vi "FA Values View.vi"(11 "Model in":refnum<class "Model.lvclass">) -> ()   [LabVIEW 2016, in "M1M3SupportEUI_Views.lvlib"]
uses:
  M1M3SupportEUI_Views.lvlib
  Model/Model.lvclass
  Typedefs/FA Data And Events.ctl
  SALLV_m1m3/DataTypes/ForceActuatorData.ctl
  SALLV_m1m3/DataTypes/logevent_ForceActuatorForceWarning.ctl
  SALLV_m1m3/DataTypes/logevent_ForceActuatorInfo.ctl
  SALLV_m1m3/DataTypes/logevent_ForceActuatorState.ctl
  SALLV_m1m3/DataTypes/logevent_ForceActuatorWarning.ctl
  SALLV_m1m3/DataTypes/logevent_AppliedAberrationForces.ctl
  SALLV_m1m3/DataTypes/logevent_AppliedAccelerationForces.ctl
  SALLV_m1m3/DataTypes/logevent_AppliedActiveOpticForces.ctl
  SALLV_m1m3/DataTypes/logevent_AppliedAzimuthForces.ctl
  SALLV_m1m3/DataTypes/logevent_AppliedBalanceForces.ctl
  SALLV_m1m3/DataTypes/logevent_AppliedCylinderForces.ctl
  SALLV_m1m3/DataTypes/logevent_AppliedElevationForces.ctl
  SALLV_m1m3/DataTypes/logevent_AppliedForces.ctl
  SALLV_m1m3/DataTypes/logevent_AppliedOffsetForces.ctl
  SALLV_m1m3/DataTypes/logevent_AppliedStaticForces.ctl
  SALLV_m1m3/DataTypes/logevent_AppliedThermalForces.ctl
  SALLV_m1m3/DataTypes/logevent_AppliedVelocityForces.ctl
  SALLV_m1m3/DataTypes/logevent_RejectedAberrationForces.ctl
  SALLV_m1m3/DataTypes/logevent_RejectedAccelerationForces.ctl
  SALLV_m1m3/DataTypes/logevent_RejectedActiveOpticForces.ctl
  SALLV_m1m3/DataTypes/logevent_RejectedAzimuthForces.ctl
  SALLV_m1m3/DataTypes/logevent_RejectedBalanceForces.ctl
  SALLV_m1m3/DataTypes/logevent_RejectedCylinderForces.ctl
  SALLV_m1m3/DataTypes/logevent_RejectedElevationForces.ctl
  SALLV_m1m3/DataTypes/logevent_RejectedForces.ctl
  SALLV_m1m3/DataTypes/logevent_RejectedOffsetForces.ctl
  SALLV_m1m3/DataTypes/logevent_RejectedStaticForces.ctl
  SALLV_m1m3/DataTypes/logevent_RejectedThermalForces.ctl
  SALLV_m1m3/DataTypes/logevent_RejectedVelocityForces.ctl
  SALLV_m1m3/DataTypes/logevent_ForceSetpointWarning.ctl
  M1M3 Support Events/M1M3 Support Events.lvclass/M1M3 Support Events.ctl
  M1M3 Support Events/M1M3 Support Events.lvclass
  <vilib>/Utility/Data Type/NI_Data Type.lvlib
  SALLV_m1m3/SALLV_m1m3.lvlib
  Typedefs/M1M3SupportEUI_TypeDefs.lvlib
panel:
  out "stop":bool
  in  "FA Data And Events":T1 {"ForceActuatorData"."Timestamp" format="%#_14f"}
  out "SingleValue":string
  out "239":string
  out "229":string
  out "219":string
  out "209":string
  out "238":string
  out "228":string
  out "218":string
  out "208":string
  out "237":string
  out "227":string
  out "217":string
  out "207":string
  out "236":string
  out "216":string
  out "235":string
  out "225":string
  out "215":string
  out "234":string
  out "224":string
  out "214":string
  out "243":string
  out "233":string
  out "223":string
  out "242":string
  out "232":string
  out "222":string
  out "212":string
  out "241":string
  out "231":string
  out "221":string
  out "211":string
  out "240":string
  out "230":string
  out "220":string
  out "210":string
  out "339":string
  out "329":string
  out "319":string
  out "309":string
  out "338":string
  out "328":string
  out "318":string
  out "308":string
  out "337":string
  out "327":string
  out "317":string
  out "307":string
  out "336":string
  out "326":string
  out "316":string
  out "306":string
  out "335":string
  out "325":string
  out "315":string
  out "305":string
  out "334":string
  out "324":string
  out "314":string
  out "304":string
  out "343":string
  out "333":string
  out "323":string
  out "313":string
  out "303":string
  out "342":string
  out "332":string
  out "322":string
  out "312":string
  out "302":string
  out "341":string
  out "331":string
  out "321":string
  out "311":string
  out "301":string
  out "340":string
  out "330":string
  out "320":string
  out "310":string
  out "439":string
  out "429":string
  out "419":string
  out "409":string
  out "438":string
  out "428":string
  out "418":string
  out "408":string
  out "437":string
  out "427":string
  out "417":string
  out "407":string
  out "436":string
  out "416":string
  out "435":string
  out "425":string
  out "415":string
  out "434":string
  out "424":string
  out "414":string
  out "443":string
  out "433":string
  out "423":string
  out "442":string
  out "432":string
  out "422":string
  out "412":string
  out "441":string
  out "431":string
  out "421":string
  out "411":string
  out "440":string
  out "430":string
  out "420":string
  out "410":string
  out "139":string
  out "129":string
  out "119":string
  out "109":string
  out "138":string
  out "128":string
  out "118":string
  out "108":string
  out "137":string
  out "127":string
  out "117":string
  out "107":string
  out "136":string
  out "126":string
  out "116":string
  out "106":string
  out "135":string
  out "125":string
  out "115":string
  out "105":string
  out "134":string
  out "124":string
  out "114":string
  out "104":string
  out "143":string
  out "133":string
  out "123":string
  out "113":string
  out "103":string
  out "142":string
  out "132":string
  out "122":string
  out "112":string
  out "102":string
  out "141":string
  out "131":string
  out "121":string
  out "111":string
  out "101":string
  out "140":string
  out "130":string
  out "120":string
  out "110":string
  out "Timestamp of Data being shown":timestamp
  in  "Data Type":string(combo)
  # "Force Actuators"
  # "0"
  # "1"
  # "2"
  # "3"
  # "4"
  # "5"
  # "6"
  # "7"
  # "8"
  # "9"
  # "100"
  # "110"
  # "120"
  # "130"
  # "140"
  # "200"
  # "210"
  # "220"
  # "230"
  # "240"
  # "300"
  # "310"
  # "320"
  # "330"
  # "340"
  # "400"
  # "410"
  # "420"
  # "430"
  # "440"
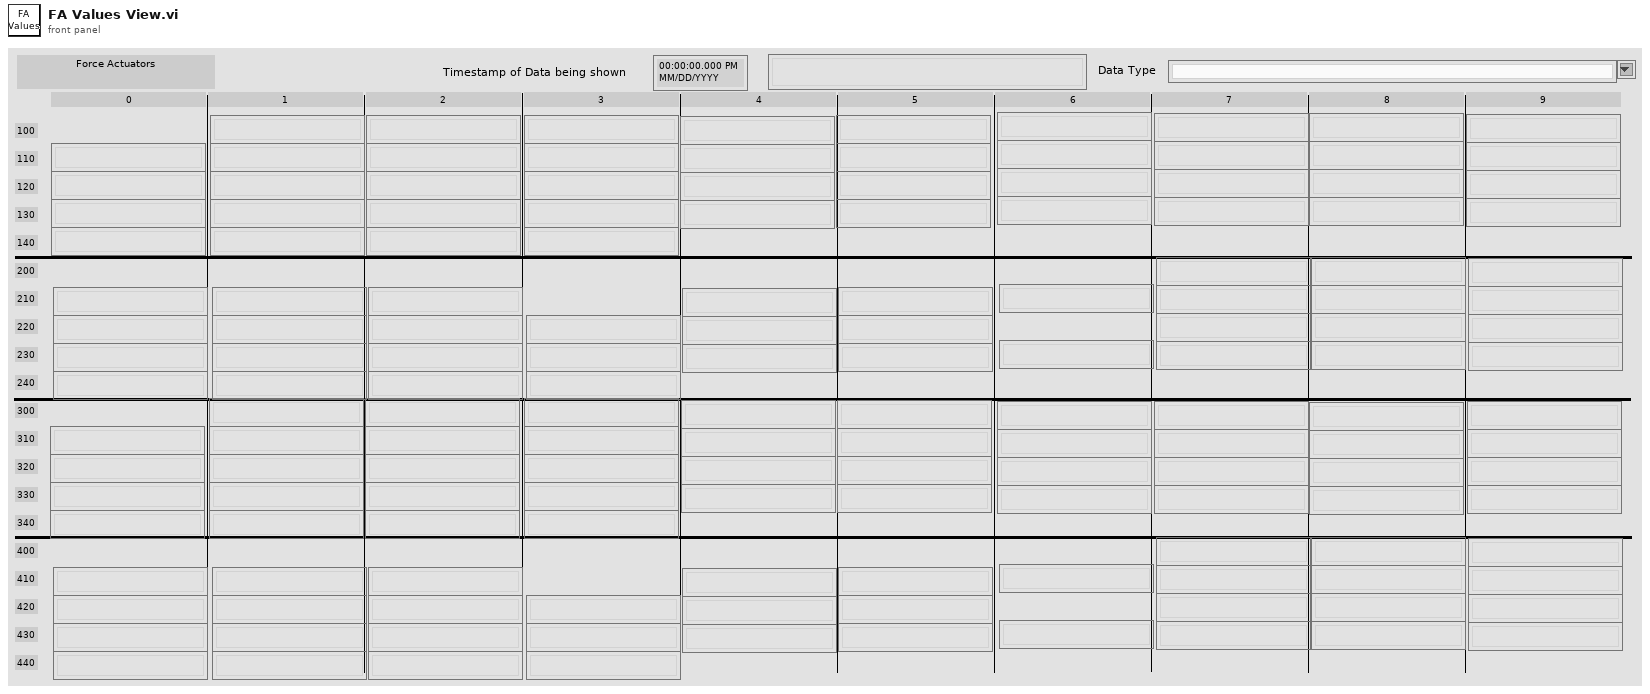
[diagram p1: front panel]
types:
  T1 = typedef "M1M3SupportEUI_TypeDefs.lvlib/FA Data And Events.ctl" = cluster{"ForceActuatorData":T2, "logevent_ForceActuatorForceWarning":T3, "logevent_ForceActuatorInfo":T4, "logevent_ForceActuatorState":T5, "logevent_ForceActuatorWarning":T6, "logevent_AppliedAberrationForces":T7, "logevent_AppliedAccelerationForces":T8, "logevent_AppliedActiveOpticForces":T9, "logevent_AppliedAzimuthForces":T10, "logevent_AppliedBalanceForces":T11, "logevent_AppliedCylinderForces":T12, "logevent_AppliedElevationForces":T13, "logevent_AppliedForces":T14, "logevent_AppliedOffsetForces":T15, "logevent_AppliedStaticForces":T16, "logevent_AppliedThermalForces":T17, "logevent_AppliedVelocityForces":T18, "logevent_RejectedAberrationForces":T19, "logevent_RejectedAccelerationForces":T20, "logevent_RejectedActiveOpticForces":T21, "logevent_RejectedAzimuthForces":T22, "logevent_RejectedBalanceForces":T23, "logevent_RejectedCylinderForces":T24, "logevent_RejectedElevationForces":T25, "logevent_RejectedForces":T26, "logevent_RejectedOffsetForces":T27, "logevent_RejectedStaticForces":T28, "logevent_RejectedThermalForces":T29, "logevent_RejectedVelocityForces":T30, "logevent_ForceSetpointWarning":T31}
  T2 = typedef "SALLV_m1m3.lvlib/ForceActuatorData.ctl" = cluster{"Timestamp":dbl, "PrimaryCylinderForce[156]":sgl[], "SecondaryCylinderForce[112]":sgl[], "XForce[12]":sgl[], "YForce[100]":sgl[], "ZForce[156]":sgl[], "Fx":sgl, "Fy":sgl, "Fz":sgl, "Mx":sgl, "My":sgl, "Mz":sgl, "ForceMagnitude":sgl}
  T3 = typedef "SALLV_m1m3.lvlib/logevent_ForceActuatorForceWarning.ctl" = cluster{"Timestamp":dbl, "AnyWarning":bool, "AnyPrimaryAxisMeasuredForceWarning":bool, "PrimaryAxisMeasuredForceWarning[156]":bool[], "AnySecondaryAxisMeasuredForceWarning":bool, "SecondaryAxisMeasuredForceWarning[156]":bool[], "AnyPrimaryAxisFollowingErrorWarning":bool, "PrimaryAxisFollowingErrorWarning[156]":bool[], "AnySecondaryAxisFollowingErrorWarning":bool, "SecondaryAxisFollowingErrorWarning[156]":bool[], "priority":i32}
  T4 = typedef "SALLV_m1m3.lvlib/logevent_ForceActuatorInfo.ctl" = cluster{"Timestamp":dbl, "ReferenceId[156]":i16[], "XDataReferenceId[12]":i16[], "YDataReferenceId[100]":i16[], "ZDataReferenceId[156]":i16[], "ActuatorType[156]":i16[], "ActuatorOrientation[156]":i16[], "ModbusSubnet[156]":i16[], "ModbusAddress[156]":i16[], "XPosition[156]":sgl[], "YPosition[156]":sgl[], "ZPosition[156]":sgl[], "ILCUniqueId[156]":i64[], "ILCApplicationType[156]":i16[], "NetworkNodeType[156]":i16[], "ILCSelectedOptions[156]":i16[], "NetworkNodeOptions[156]":i16[], "MajorRevision[156]":i16[], "MinorRevision[156]":i16[], "ADCScanRate[156]":i16[], "MainPrimaryCylinderCoefficient[156]":sgl[], "MainSecondaryCylinderCoefficient[156]":sgl[], "MainPrimaryCylinderLoadCellOffset[156]":sgl[], "MainSecondaryCylinderLoadCellOffset[156]":sgl[], "MainPrimaryCylinderLoadCellSensitivity[156]":sgl[], "MainSecondaryCylinderLoadCellSensitivity[156]":sgl[], "BackupPrimaryCylinderCoefficient[156]":sgl[], "BackupSecondaryCylinderCoefficient[156]":sgl[], "BackupPrimaryCylinderLoadCellOffset[156]":sgl[], "BackupSecondaryCylinderLoadCellOffset[156]":sgl[], "BackupPrimaryCylinderLoadCellSensitivity[156]":sgl[], "BackupSecondaryCylinderLoadCellSensitivity[156]":sgl[], "MezzaninePrimaryCylinderGain[156]":sgl[], "MezzanineSecondaryCylinderGain[156]":sgl[], "MezzanineUniqueId[156]":i64[], "MezzanineFirmwareType[156]":i16[], "MezzanineMajorRevision[156]":i16[], "MezzanineMinorRevision[156]":i16[], "priority":i32}
  T5 = typedef "SALLV_m1m3.lvlib/logevent_ForceActuatorState.ctl" = cluster{"Timestamp":dbl, "ILCState[156]":i16[], "SlewFlag":bool, "StaticForcesApplied":bool, "ElevationForcesApplied":bool, "AzimuthForcesApplied":bool, "ThermalForcesApplied":bool, "OffsetForcesApplied":bool, "AccelerationForcesApplied":bool, "VelocityForcesApplied":bool, "ActiveOpticForcesApplied":bool, "AberrationForcesApplied":bool, "BalanceForcesApplied":bool, "SupportPercentage":sgl, "priority":i32}
  T6 = typedef "SALLV_m1m3.lvlib/logevent_ForceActuatorWarning.ctl" = cluster{"Timestamp":dbl, "AnyWarning":bool, "AnyMajorFault":bool, "MajorFault[156]":bool[], "AnyMinorFault":bool, "MinorFault[156]":bool[], "AnyFaultOverride":bool, "FaultOverride[156]":bool[], "AnyMainCalibrationError":bool, "MainCalibrationError[156]":bool[], "AnyBackupCalibrationError":bool, "BackupCalibrationError[156]":bool[], "AnyMezzanineError":bool, "MezzanineError[156]":bool[], "AnyMezzanineBootloaderActive":bool, "MezzanineBootloaderActive[156]":bool[], "AnyUniqueIdCRCError":bool, "UniqueIdCRCError[156]":bool[], "AnyApplicationTypeMismatch":bool, "ApplicationTypeMismatch[156]":bool[], "AnyApplicationMissing":bool, "ApplicationMissing[156]":bool[], "AnyApplicationCRCMismatch":bool, "ApplicationCRCMismatch[156]":bool[], "AnyOneWireMissing":bool, "OneWireMissing[156]":bool[], "AnyOneWire1Mismatch":bool, "OneWire1Mismatch[156]":bool[], "AnyOneWire2Mismatch":bool, "OneWire2Mismatch[156]":bool[], "AnyWatchdogReset":bool, "WatchdogReset[156]":bool[], "AnyBrownOut":bool, "BrownOut[156]":bool[], "AnyEventTrapReset":bool, "EventTrapReset[156]":bool[], "AnySSRPowerFault":bool, "SSRPowerFault[156]":bool[], "AnyAuxPowerFault":bool, "AuxPowerFault[156]":bool[], "AnyMezzaninePowerFault":bool, "MezzaninePowerFault[156]":bool[], "AnyMezzanineCurrentAmp1Fault":bool, "MezzanineCurrentAmp1Fault[156]":bool[], "AnyMezzanineCurrentAmp2Fault":bool, "MezzanineCurrentAmp2Fault[156]":bool[], "AnyMezzanineUniqueIdCRCError":bool, "MezzanineUniqueIdCRCError[156]":bool[], "AnyMezzanineMainCalibrationError":bool, "MezzanineMainCalibrationError[156]":bool[], "AnyMezzanineBackupCalibrationError":bool, "MezzanineBackupCalibrationError[156]":bool[], "AnyMezzanineEventTrapReset":bool, "MezzanineEventTrapReset[156]":bool[], "AnyMezzanineApplicationMissing":bool, "MezzanineApplicationMissing[156]":bool[], "AnyMezzanineApplicationCRCMismatch":bool, "MezzanineApplicationCRCMismatch[156]":bool[], "AnyILCFault":bool, "ILCFault[156]":bool[], "AnyBroadcastCounterWarning":bool, "BroadcastCounterWarning[156]":bool[], "priority":i32}
  T7 = typedef "SALLV_m1m3.lvlib/logevent_AppliedAberrationForces.ctl" = cluster{"Timestamp":dbl, "ZForces[156]":sgl[], "Fz":sgl, "Mx":sgl, "My":sgl, "priority":i32}
  T8 = typedef "SALLV_m1m3.lvlib/logevent_AppliedAccelerationForces.ctl" = cluster{"Timestamp":dbl, "XForces[12]":sgl[], "YForces[100]":sgl[], "ZForces[156]":sgl[], "Fx":sgl, "Fy":sgl, "Fz":sgl, "Mx":sgl, "My":sgl, "Mz":sgl, "ForceMagnitude":sgl, "priority":i32}
  T9 = typedef "SALLV_m1m3.lvlib/logevent_AppliedActiveOpticForces.ctl" = cluster{"Timestamp":dbl, "ZForces[156]":sgl[], "Fz":sgl, "Mx":sgl, "My":sgl, "priority":i32}
  T10 = typedef "SALLV_m1m3.lvlib/logevent_AppliedAzimuthForces.ctl" = cluster{"Timestamp":dbl, "XForces[12]":sgl[], "YForces[100]":sgl[], "ZForces[156]":sgl[], "Fx":sgl, "Fy":sgl, "Fz":sgl, "Mx":sgl, "My":sgl, "Mz":sgl, "ForceMagnitude":sgl, "priority":i32}
  T11 = typedef "SALLV_m1m3.lvlib/logevent_AppliedBalanceForces.ctl" = cluster{"Timestamp":dbl, "XForces[12]":sgl[], "YForces[100]":sgl[], "ZForces[156]":sgl[], "Fx":sgl, "Fy":sgl, "Fz":sgl, "Mx":sgl, "My":sgl, "Mz":sgl, "ForceMagnitude":sgl, "priority":i32}
  T12 = typedef "SALLV_m1m3.lvlib/logevent_AppliedCylinderForces.ctl" = cluster{"Timestamp":dbl, "SecondaryCylinderForces[112]":i32[], "PrimaryCylinderForces[156]":i32[], "priority":i32}
  T13 = typedef "SALLV_m1m3.lvlib/logevent_AppliedElevationForces.ctl" = cluster{"Timestamp":dbl, "XForces[12]":sgl[], "YForces[100]":sgl[], "ZForces[156]":sgl[], "Fx":sgl, "Fy":sgl, "Fz":sgl, "Mx":sgl, "My":sgl, "Mz":sgl, "ForceMagnitude":sgl, "priority":i32}
  T14 = typedef "SALLV_m1m3.lvlib/logevent_AppliedForces.ctl" = cluster{"Timestamp":dbl, "XForces[12]":sgl[], "YForces[100]":sgl[], "ZForces[156]":sgl[], "Fx":sgl, "Fy":sgl, "Fz":sgl, "Mx":sgl, "My":sgl, "Mz":sgl, "ForceMagnitude":sgl, "priority":i32}
  T15 = typedef "SALLV_m1m3.lvlib/logevent_AppliedOffsetForces.ctl" = cluster{"Timestamp":dbl, "XForces[12]":sgl[], "YForces[100]":sgl[], "ZForces[156]":sgl[], "Fx":sgl, "Fy":sgl, "Fz":sgl, "Mx":sgl, "My":sgl, "Mz":sgl, "ForceMagnitude":sgl, "priority":i32}
  T16 = typedef "SALLV_m1m3.lvlib/logevent_AppliedStaticForces.ctl" = cluster{"Timestamp":dbl, "XForces[12]":sgl[], "YForces[100]":sgl[], "ZForces[156]":sgl[], "Fx":sgl, "Fy":sgl, "Fz":sgl, "Mx":sgl, "My":sgl, "Mz":sgl, "ForceMagnitude":sgl, "priority":i32}
  T17 = typedef "SALLV_m1m3.lvlib/logevent_AppliedThermalForces.ctl" = cluster{"Timestamp":dbl, "XForces[12]":sgl[], "YForces[100]":sgl[], "ZForces[156]":sgl[], "Fx":sgl, "Fy":sgl, "Fz":sgl, "Mx":sgl, "My":sgl, "Mz":sgl, "ForceMagnitude":sgl, "priority":i32}
  T18 = typedef "SALLV_m1m3.lvlib/logevent_AppliedVelocityForces.ctl" = cluster{"Timestamp":dbl, "XForces[12]":sgl[], "YForces[100]":sgl[], "ZForces[156]":sgl[], "Fx":sgl, "Fy":sgl, "Fz":sgl, "Mx":sgl, "My":sgl, "Mz":sgl, "ForceMagnitude":sgl, "priority":i32}
  T19 = typedef "SALLV_m1m3.lvlib/logevent_RejectedAberrationForces.ctl" = cluster{"Timestamp":dbl, "ZForces[156]":sgl[], "Fz":sgl, "Mx":sgl, "My":sgl, "priority":i32}
  T20 = typedef "SALLV_m1m3.lvlib/logevent_RejectedAccelerationForces.ctl" = cluster{"Timestamp":dbl, "XForces[12]":sgl[], "YForces[100]":sgl[], "ZForces[156]":sgl[], "Fx":sgl, "Fy":sgl, "Fz":sgl, "Mx":sgl, "My":sgl, "Mz":sgl, "ForceMagnitude":sgl, "priority":i32}
  T21 = typedef "SALLV_m1m3.lvlib/logevent_RejectedActiveOpticForces.ctl" = cluster{"Timestamp":dbl, "ZForces[156]":sgl[], "Fz":sgl, "Mx":sgl, "My":sgl, "priority":i32}
  T22 = typedef "SALLV_m1m3.lvlib/logevent_RejectedAzimuthForces.ctl" = cluster{"Timestamp":dbl, "XForces[12]":sgl[], "YForces[100]":sgl[], "ZForces[156]":sgl[], "Fx":sgl, "Fy":sgl, "Fz":sgl, "Mx":sgl, "My":sgl, "Mz":sgl, "ForceMagnitude":sgl, "priority":i32}
  T23 = typedef "SALLV_m1m3.lvlib/logevent_RejectedBalanceForces.ctl" = cluster{"Timestamp":dbl, "XForces[12]":sgl[], "YForces[100]":sgl[], "ZForces[156]":sgl[], "Fx":sgl, "Fy":sgl, "Fz":sgl, "Mx":sgl, "My":sgl, "Mz":sgl, "ForceMagnitude":sgl, "priority":i32}
  T24 = typedef "SALLV_m1m3.lvlib/logevent_RejectedCylinderForces.ctl" = cluster{"Timestamp":dbl, "SecondaryCylinderForces[112]":i32[], "PrimaryCylinderForces[156]":i32[], "priority":i32}
  T25 = typedef "SALLV_m1m3.lvlib/logevent_RejectedElevationForces.ctl" = cluster{"Timestamp":dbl, "XForces[12]":sgl[], "YForces[100]":sgl[], "ZForces[156]":sgl[], "Fx":sgl, "Fy":sgl, "Fz":sgl, "Mx":sgl, "My":sgl, "Mz":sgl, "ForceMagnitude":sgl, "priority":i32}
  T26 = typedef "SALLV_m1m3.lvlib/logevent_RejectedForces.ctl" = cluster{"Timestamp":dbl, "XForces[12]":sgl[], "YForces[100]":sgl[], "ZForces[156]":sgl[], "Fx":sgl, "Fy":sgl, "Fz":sgl, "Mx":sgl, "My":sgl, "Mz":sgl, "ForceMagnitude":sgl, "priority":i32}
  T27 = typedef "SALLV_m1m3.lvlib/logevent_RejectedOffsetForces.ctl" = cluster{"Timestamp":dbl, "XForces[12]":sgl[], "YForces[100]":sgl[], "ZForces[156]":sgl[], "Fx":sgl, "Fy":sgl, "Fz":sgl, "Mx":sgl, "My":sgl, "Mz":sgl, "ForceMagnitude":sgl, "priority":i32}
  T28 = typedef "SALLV_m1m3.lvlib/logevent_RejectedStaticForces.ctl" = cluster{"Timestamp":dbl, "XForces[12]":sgl[], "YForces[100]":sgl[], "ZForces[156]":sgl[], "Fx":sgl, "Fy":sgl, "Fz":sgl, "Mx":sgl, "My":sgl, "Mz":sgl, "ForceMagnitude":sgl, "priority":i32}
  T29 = typedef "SALLV_m1m3.lvlib/logevent_RejectedThermalForces.ctl" = cluster{"Timestamp":dbl, "XForces[12]":sgl[], "YForces[100]":sgl[], "ZForces[156]":sgl[], "Fx":sgl, "Fy":sgl, "Fz":sgl, "Mx":sgl, "My":sgl, "Mz":sgl, "ForceMagnitude":sgl, "priority":i32}
  T30 = typedef "SALLV_m1m3.lvlib/logevent_RejectedVelocityForces.ctl" = cluster{"Timestamp":dbl, "XForces[12]":sgl[], "YForces[100]":sgl[], "ZForces[156]":sgl[], "Fx":sgl, "Fy":sgl, "Fz":sgl, "Mx":sgl, "My":sgl, "Mz":sgl, "ForceMagnitude":sgl, "priority":i32}
  T31 = typedef "SALLV_m1m3.lvlib/logevent_ForceSetpointWarning.ctl" = cluster{"Timestamp":dbl, "AnyWarning":bool, "AnySafetyLimitWarning":bool, "SafetyLimitWarning[156]":bool[], "XMomentWarning":bool, "YMomentWarning":bool, "ZMomentWarning":bool, "AnyNearNeighborWarning":bool, "NearNeighborWarning[156]":bool[], "MagnitudeWarning":bool, "AnyFarNeighborWarning":bool, "FarNeighborWarning[156]":bool[], "AnyElevationForceWarning":bool, "ElevationForceWarning[156]":bool[], "AnyAzimuthForceWarning":bool, "AzimuthForceWarning[156]":bool[], "AnyThermalForceWarning":bool, "ThermalForceWarning[156]":bool[], "AnyBalanceForceWarning":bool, "BalanceForceWarning[156]":bool[], "AnyAccelerationForceWarning":bool, "AccelerationForceWarning[156]":bool[], "ActiveOpticNetForceWarning":bool, "AnyActiveOpticForceWarning":bool, "ActiveOpticForceWarning[156]":bool[], "AnyStaticForceWarning":bool, "StaticForceWarning[156]":bool[], "AberrationNetForceWarning":bool, "AnyAberrationForceWarning":bool, "AberrationForceWarning[156]":bool[], "AnyOffsetForceWarning":bool, "OffsetForceWarning[156]":bool[], "AnyVelocityForceWarning":bool, "VelocityForceWarning[156]":bool[], "AnyForceWarning":bool, "ForceWarning[156]":bool[], "priority":i32}
  T32 = typedef "M1M3SupportEUI_TypeDefs.lvlib/M1M3 Support Events.ctl" = cluster{"Inclinometer  Data":refnum<user-event>, "IMS Data":refnum<user-event>, "SAL Connected":refnum<user-event>, "Accelerometer Data":refnum<user-event>, "OuterLoop Data":refnum<user-event>, "ErrorCode Event":refnum<user-event>, "InterlockStatus Event":refnum<user-event>, "InterlockWarning Event":refnum<user-event>, "Gyro Data":refnum<user-event>, "HP Actuator Info Event":refnum<user-event>, " FA Info Event":refnum<user-event>, "HP Monitor Info Event":refnum<user-event>, "FA Data":refnum<user-event>, "HP Actuator data":refnum<user-event>, "HP Monitor data":refnum<user-event>, "Air Supply Status Event":refnum<user-event>, "Air Supply Warning Event":refnum<user-event>, "Power Data":refnum<user-event>, "PID Data":refnum<user-event>, "PID Info Event":refnum<user-event>, "Power Status Event":refnum<user-event>, "Power Supply Status Event":refnum<user-event>, "Power Warning Event":refnum<user-event>, "Summary State Event":refnum<user-event>, "Detailed State Event":refnum<user-event>, "FA Force Warning Event":refnum<user-event>, "FA Warning Event":refnum<user-event>, "FA State Event":refnum<user-event>, "Applied AberrationForces Event":refnum<user-event>, "Applied Acceleration Forcces Event":refnum<user-event>, "Applied Azimuth Forces Event":refnum<user-event>, "Applied Active Optic Forces Event":refnum<user-event>, "Applied Balance Forces Event":refnum<user-event>, "Applied Cylinder Forces Event":refnum<user-event>, "Applied Elevation Forces Event":refnum<user-event>, "Applied Forces Event":refnum<user-event>, "Applied Offset Forces Event":refnum<user-event>, "Applied Static Forces Event":refnum<user-event>, "Applied Thermal Forces Event":refnum<user-event>, "Applied Velocity Forces Event":refnum<user-event>, "Rejected Aberration Force Event":refnum<user-event>, "Rejected Acceleration Forces Event":refnum<user-event>, "Rejected Active Optic Forces Event":refnum<user-event>, "Rejected Azimuth Forces Event":refnum<user-event>, "Rejected Balance Forces Event":refnum<user-event>, "Rejected Cylinder Forces Event":refnum<user-event>, "Rejected Elevation Forces Event":refnum<user-event>, "Rejected Forces Event":refnum<user-event>, "Rejected Offset Forces Event":refnum<user-event>, "Rejected Static Forces Event":refnum<user-event>, "Rejected Thermal Forces Event":refnum<user-event>, "Rejected Velocity Forces Event":refnum<user-event>, "Command Rejection Event":refnum<user-event>, "Setting Verions Event":refnum<user-event>, "Settings Applied Event":refnum<user-event>, "HP Actuator State Event":refnum<user-event>, "HP Actuator Warning Event":refnum<user-event>, "HP Monitor State Event":refnum<user-event>, "HP Monitor Warning Event":refnum<user-event>, "Accelerometer Warning Event":refnum<user-event>, "Applied Settings Match Start Event":refnum<user-event>, "Cell Light Status Event ":refnum<user-event>, "Cell Light Warning Event":refnum<user-event>, "Displacement Sensor Warning Event":refnum<user-event>, "Force Setpoint Warning Event":refnum<user-event>, "Gyro Warning Event ":refnum<user-event>, "ILC Warning Event ":refnum<user-event>, "Inclinometer Sensor Warning Event ":refnum<user-event>}
  T33 = typedef "NI_Data Type.lvlib/Data Type.ctl" = enum8{"Invalid Type", "Void", "I8", "I16", "I32", "I64", "U8", "U16", "U32", "U64", "Single Float", "Double Float", "Extended Float", "Single Complex", "Double Complex", "Extended Complex", "Enum U8", "Enum U16", "Enum U32", "Enum U64", "Single Float With Unit", "Double Float With Unit", "Extended Float With Unit", "Single Complex with Unit", "Double Complex with Unit", "Extended Complex with Unit", "Boolean", "String", "Path", "Picture", "Tag", "Array", "Cluster", "Variant", "LV Variant", "Waveform", "Timestamp", "Digital Waveform", "Digital Data", "ExpressData", "Refnum", "External Data", "VI", "Poly VI", "LabVIEW Class Instance", "Fixed Point"}
  T34 = enum16{"", "DetailedState_DetailedStates_DisabledState", "DetailedState_DetailedStates_EnabledState", "DetailedState_DetailedStates_FaultState", "DetailedState_DetailedStates_OfflineState", "DetailedState_DetailedStates_StandbyState", "DetailedState_DetailedStates_ParkedState", "DetailedState_DetailedStates_RaisingState", "DetailedState_DetailedStates_ActiveState", "DetailedState_DetailedStates_LoweringState", "DetailedState_DetailedStates_EngineeringState", "DetailedState_DetailedStates_ParkedEngineeringState", "DetailedState_DetailedStates_RaisingEngineeringState", "DetailedState_DetailedStates_ActiveEngineeringState", "DetailedState_DetailedStates_LoweringEngineeringState", "DetailedState_DetailedStates_LoweringFaultState", "DetailedState_DetailedStates_ProfileHardpointCorrectionState"}
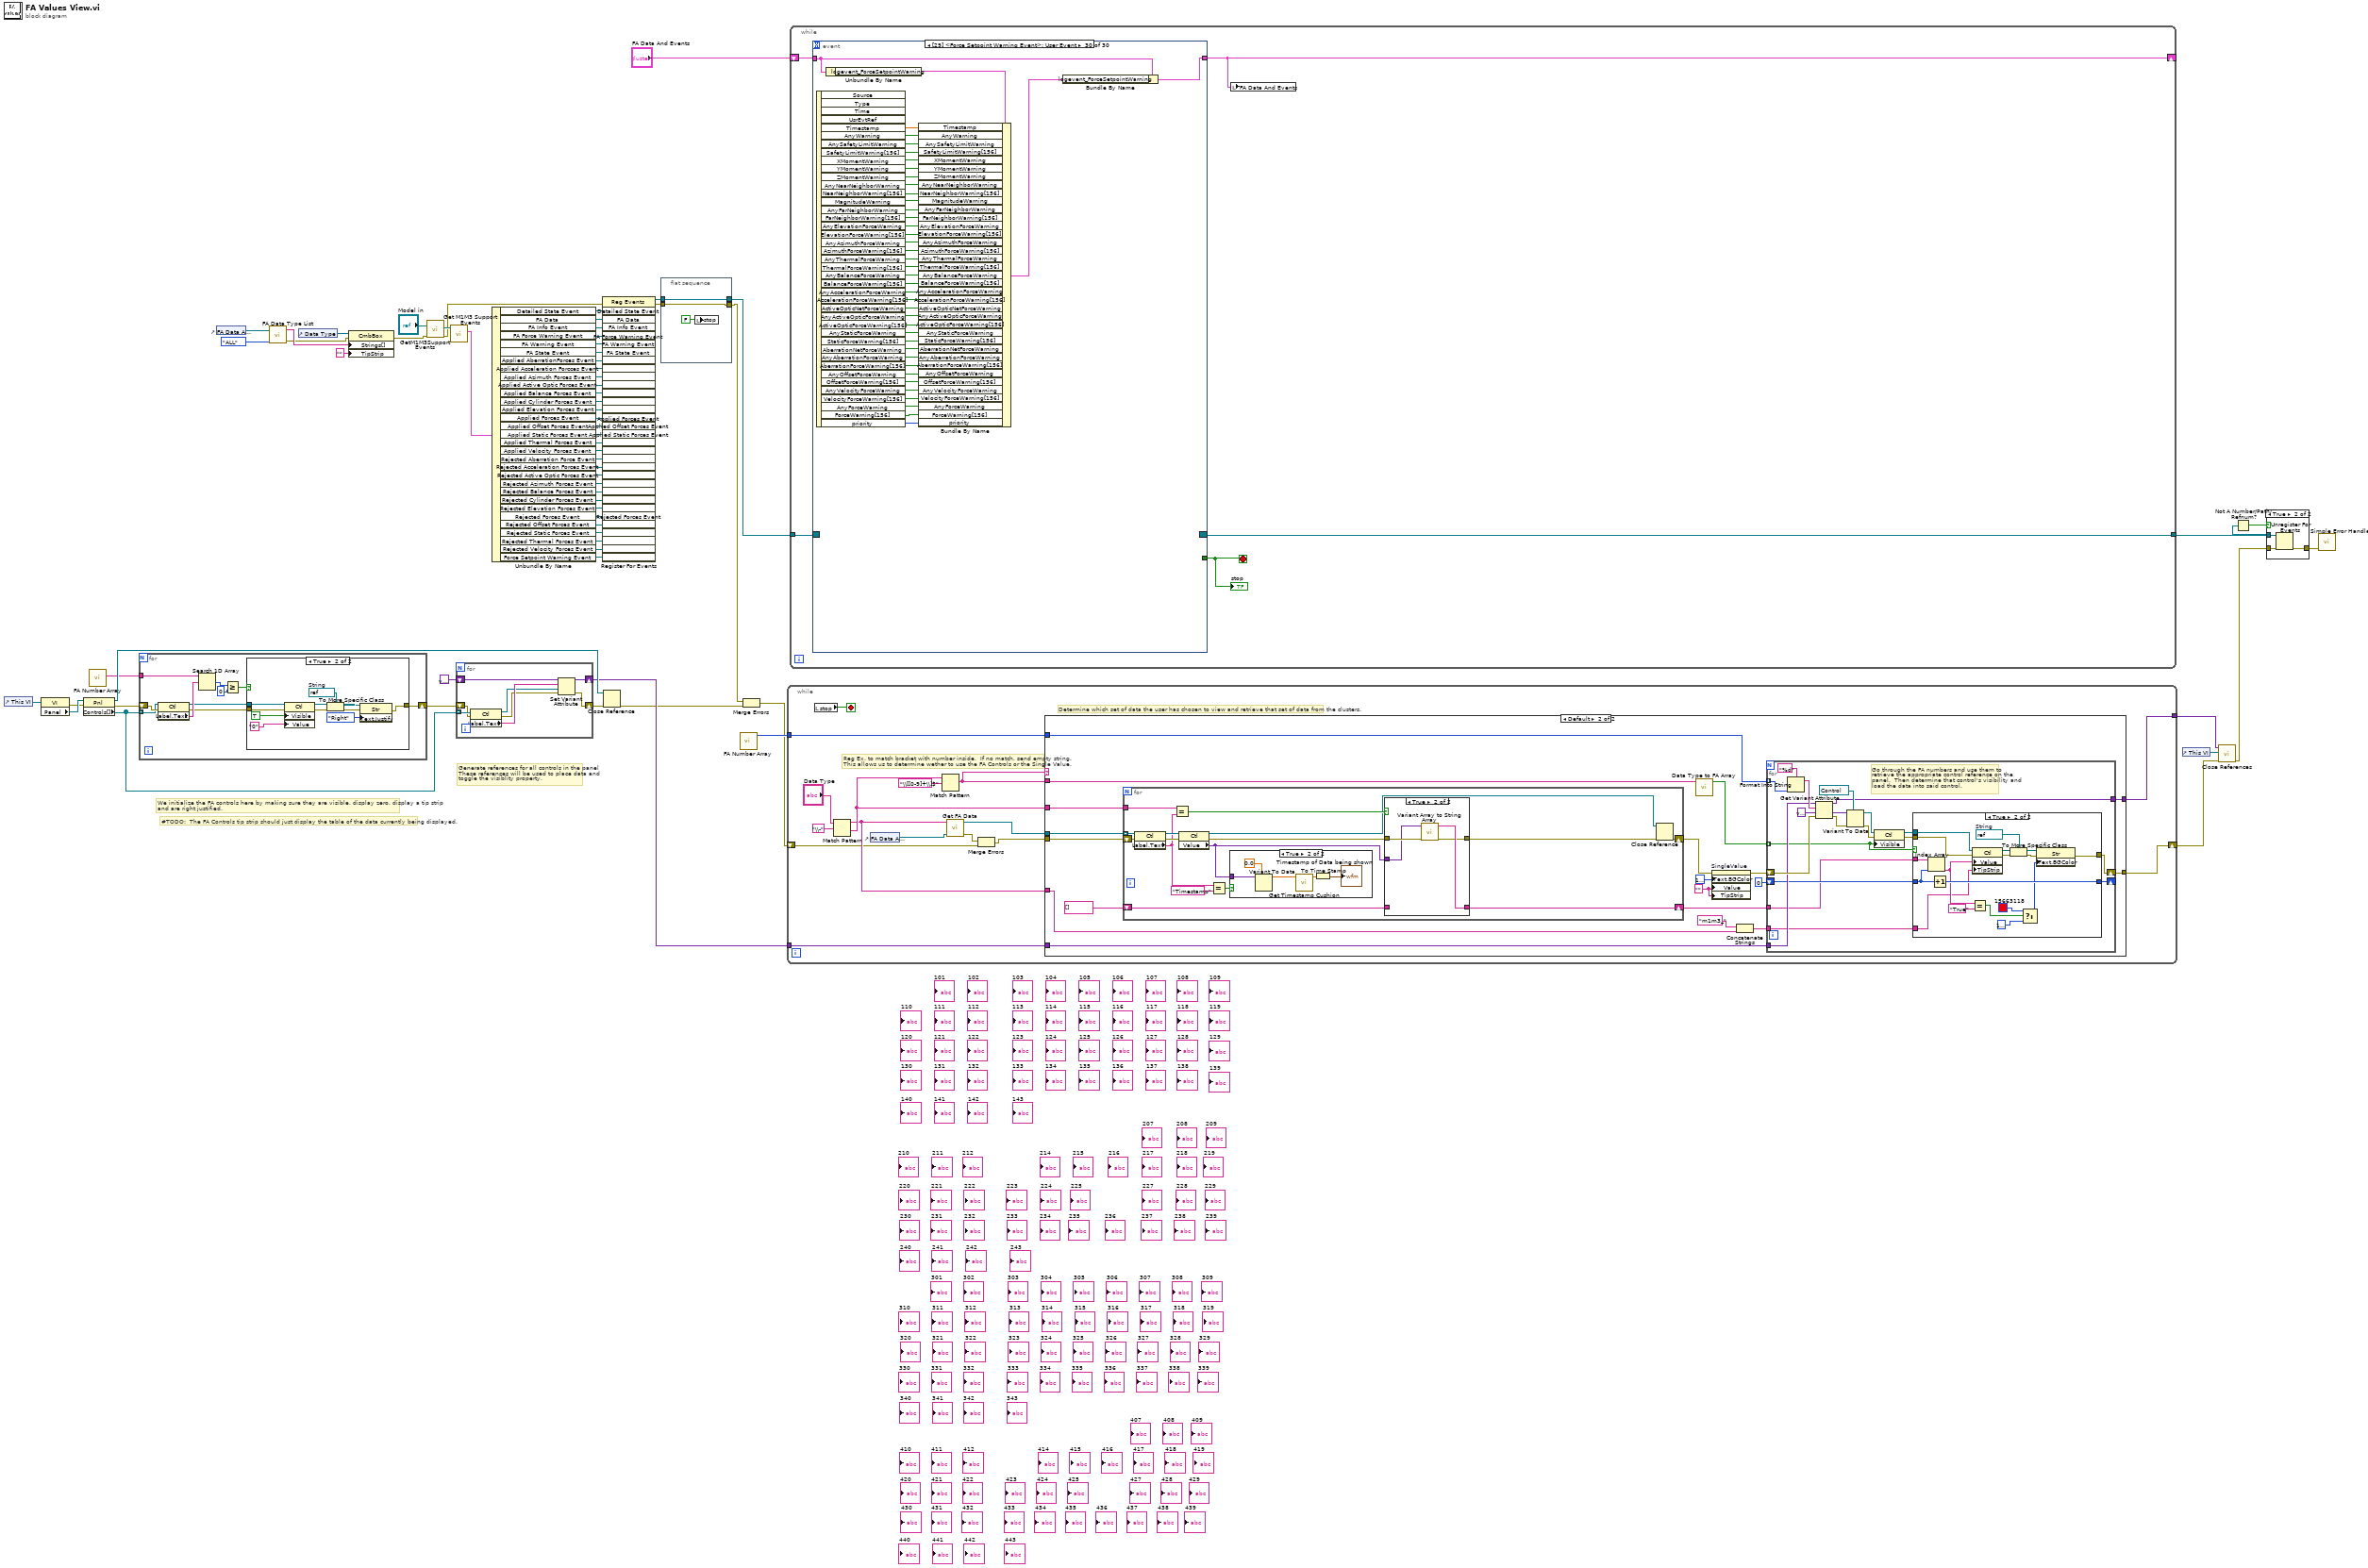
[diagram p0: block diagram]
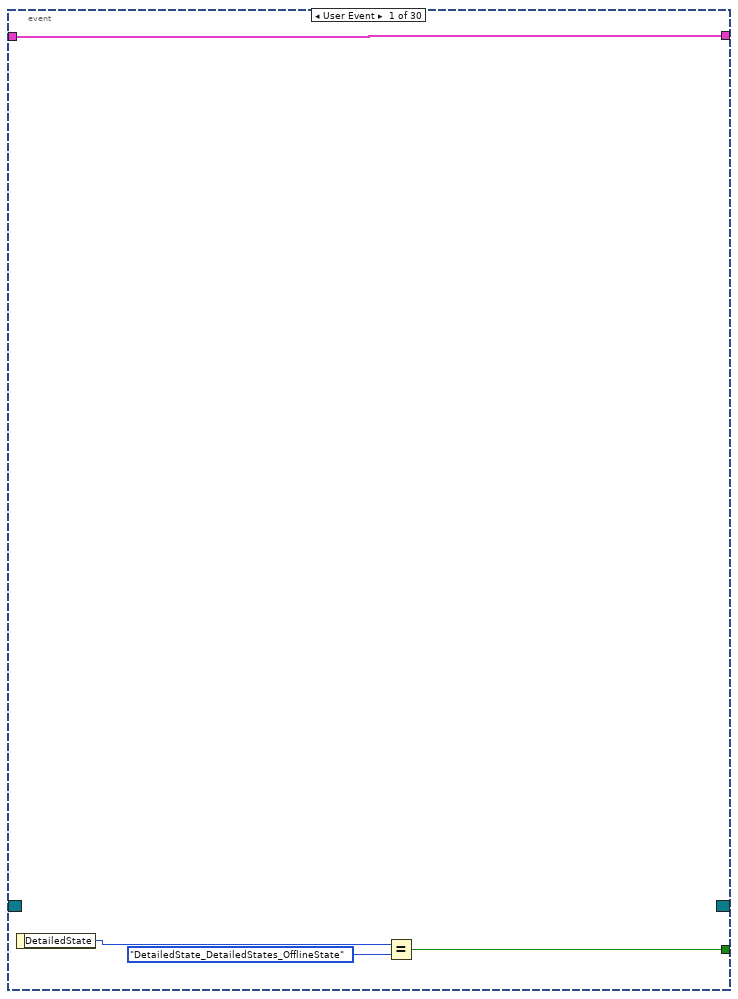
[diagram p3: hidden frame]
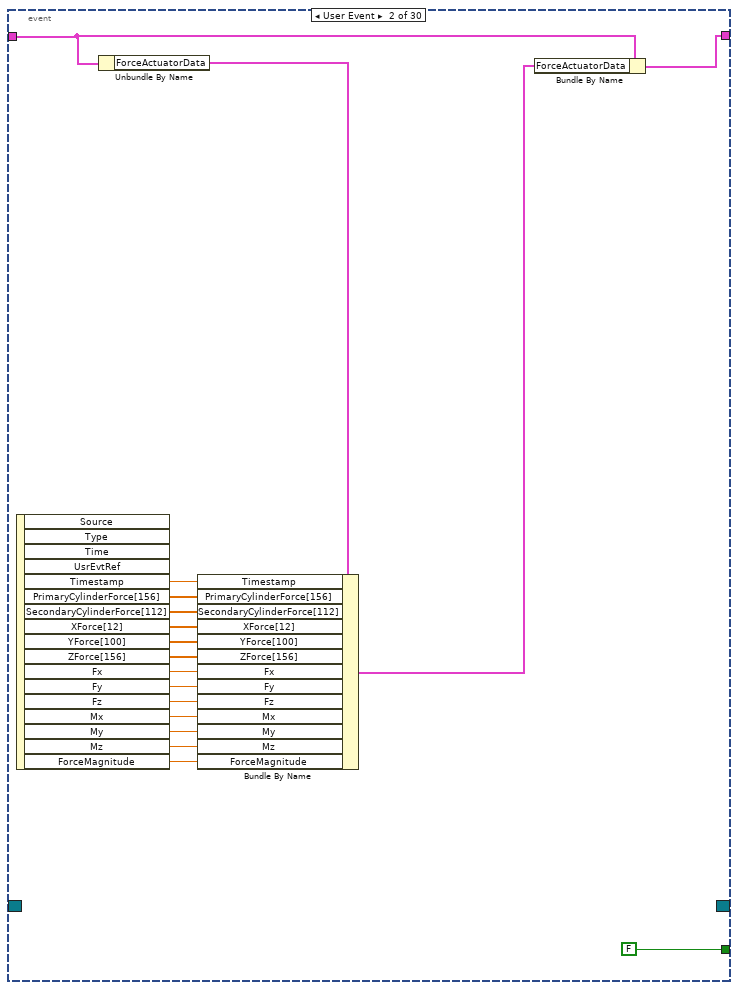
[diagram p4: hidden frame]
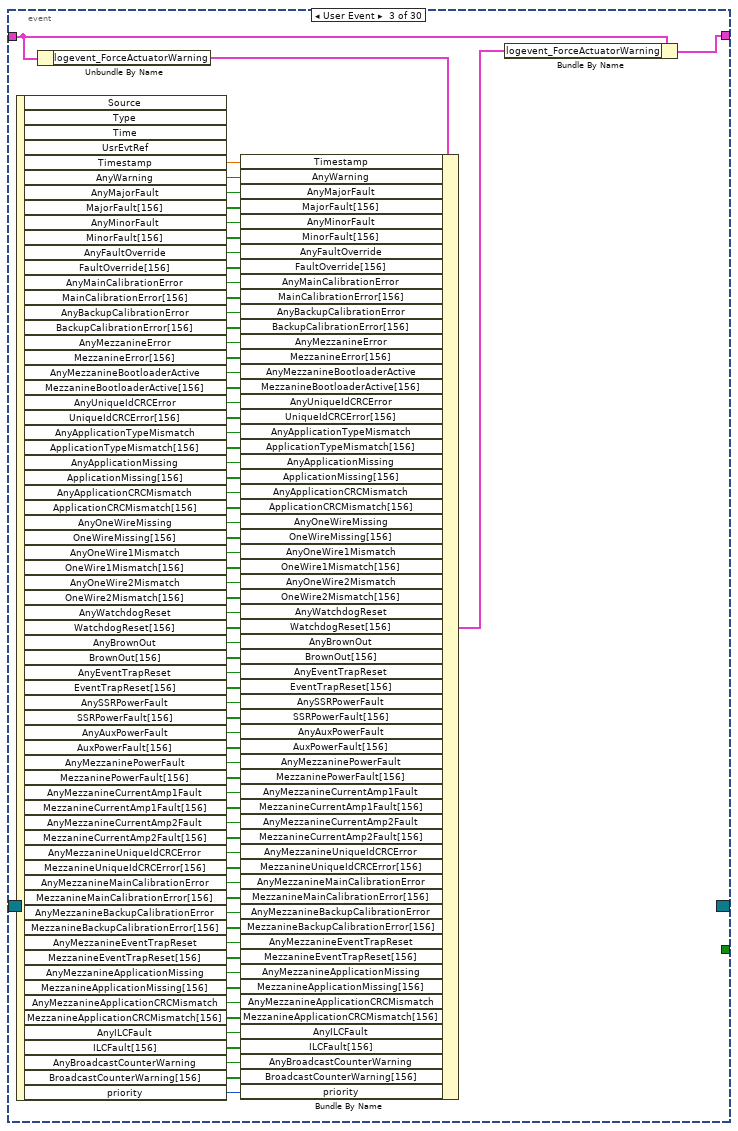
[diagram p5: hidden frame]
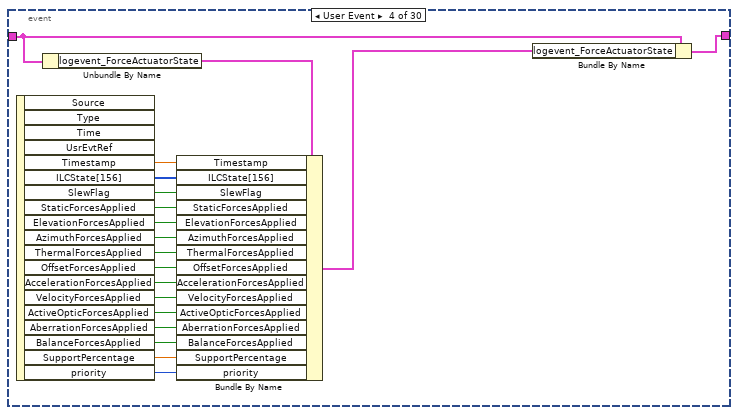
[diagram p6: hidden frame]
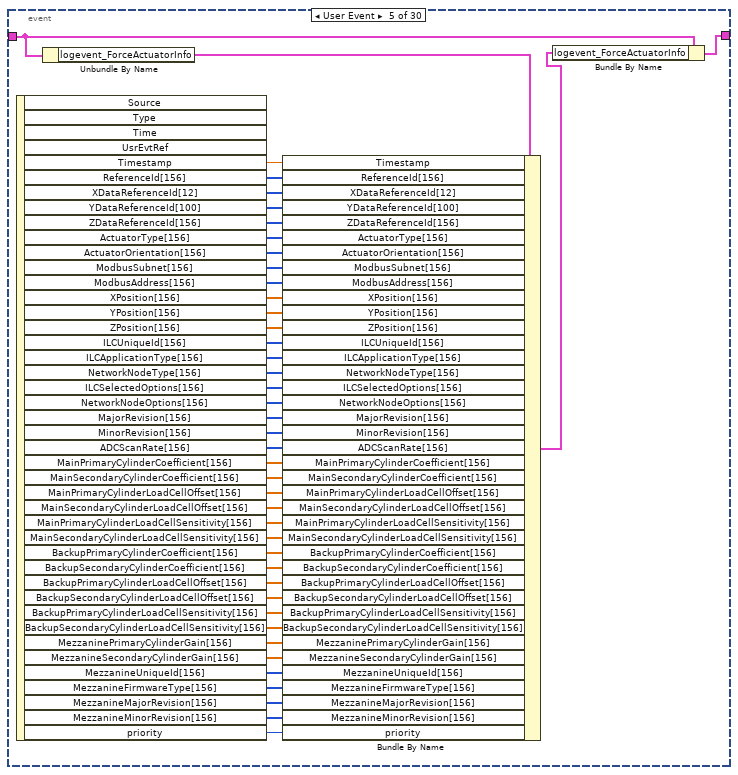
[diagram p7: hidden frame]
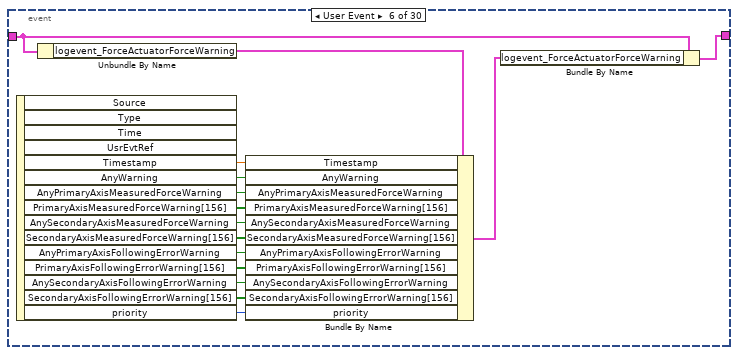
[diagram p8: hidden frame]
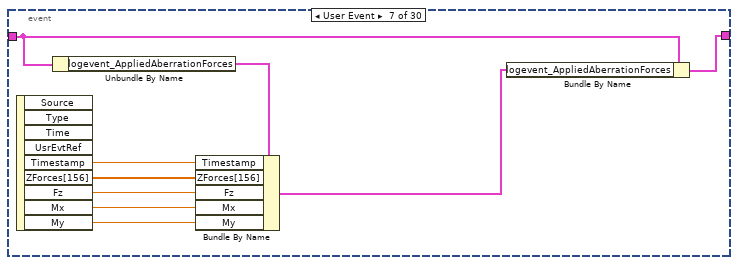
[diagram p9: hidden frame]
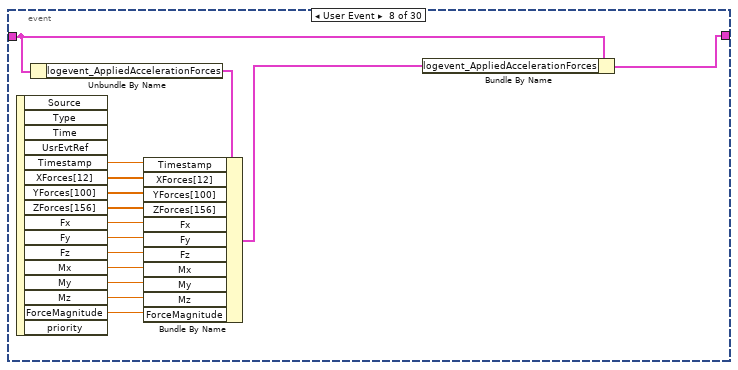
[diagram p10: hidden frame]
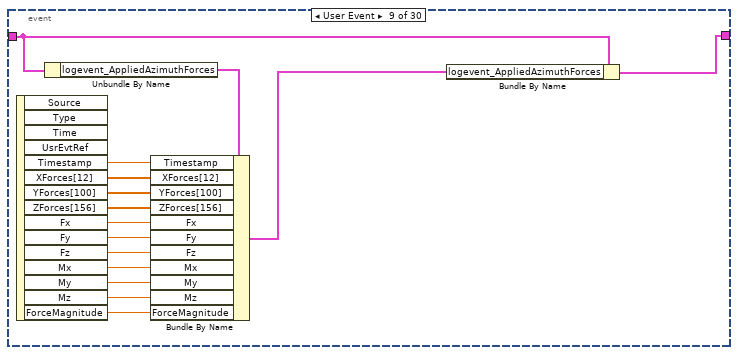
[diagram p11: hidden frame]
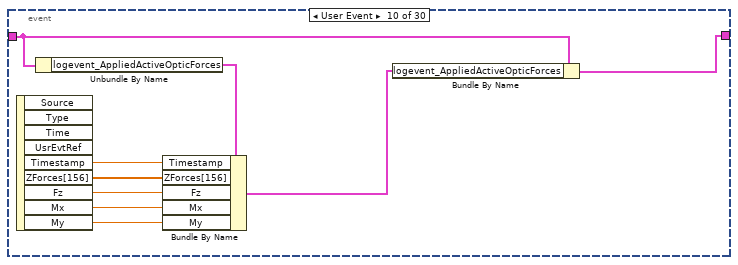
[diagram p12: hidden frame]
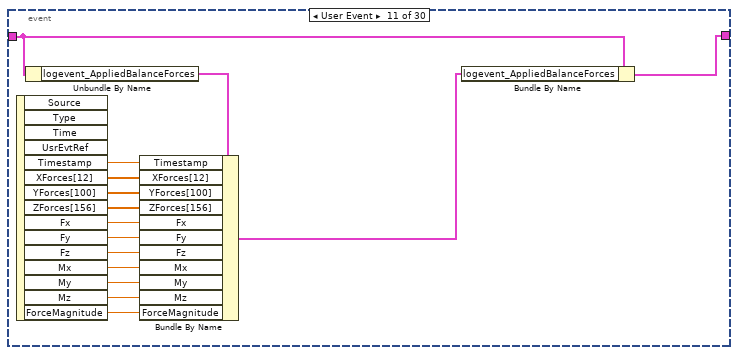
[diagram p13: hidden frame]
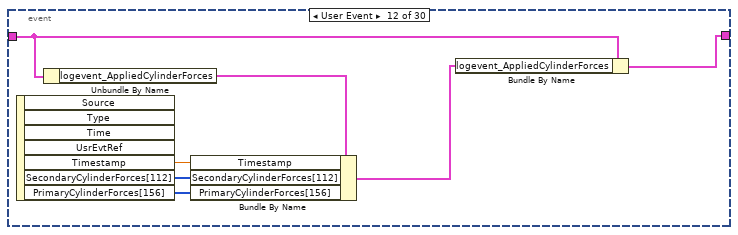
[diagram p14: hidden frame]
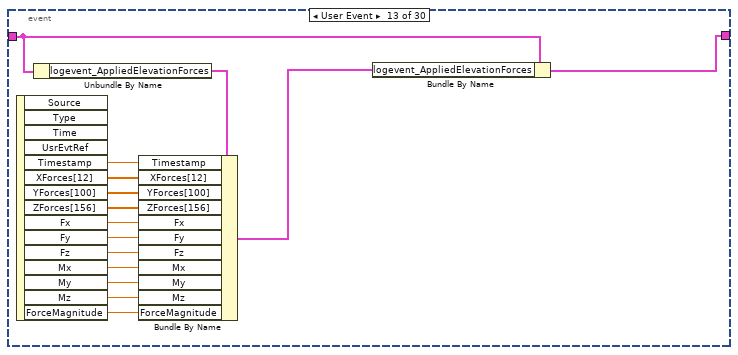
[diagram p15: hidden frame]
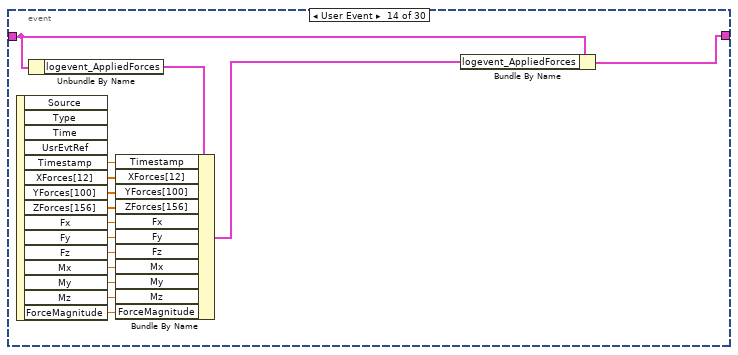
[diagram p16: hidden frame]
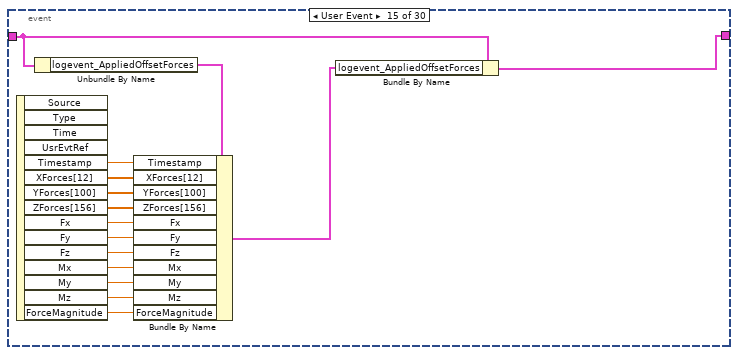
[diagram p17: hidden frame]
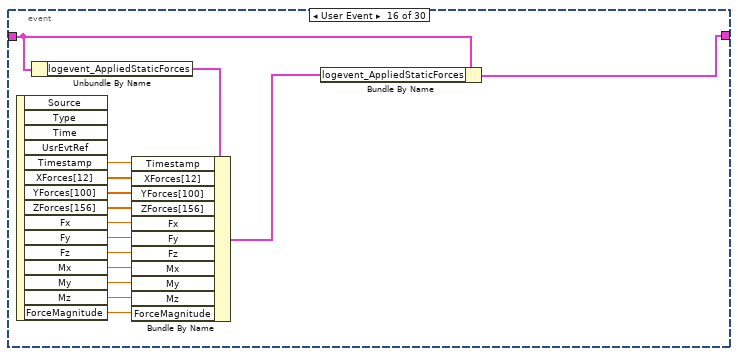
[diagram p18: hidden frame]
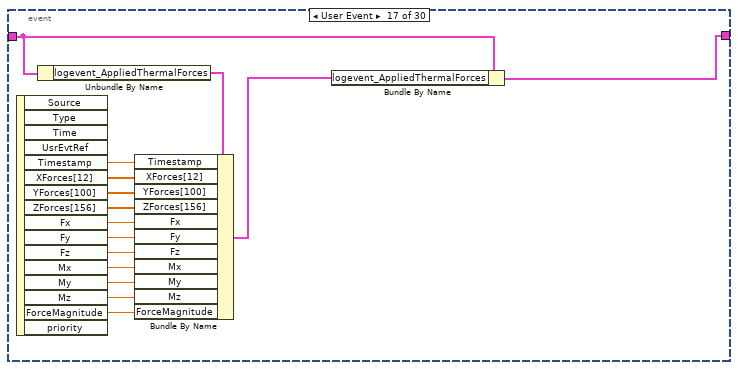
[diagram p19: hidden frame]
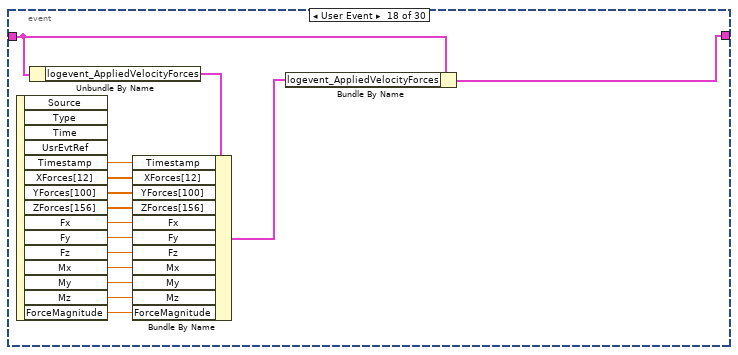
[diagram p20: hidden frame]
diagram:
  # "#TODO:  The FA Controls tip strip should just display the table of the data currently being displayed."
  # "We initialize the FA controls here by making sure they are visible, display zero, display a tip strip\nand are right justified."
  # "Generate references for all controls in the panel\nThese references will be used to place data and\ntoggle the visiblity property."
  n1 = control-ref of="This VI"() -> (w53:refnum<vi>)
  n2 = property class="VI"(reference=w53) -> (error out=w54:errorcluster, "Panel"=w55:refnum<vi>)  [unwired: 1 in, 1 out]
  n3 = property class="Pnl"(reference=w55, error in=w54) -> (reference out=w50:refnum<vi>, error out=w56:errorcluster, "Controls[]"=w52:refnum<vi>[])
  n4 = call "FA Number Array.vi"() -> ("FA Number String Array"=w49:string[])  [unwired: 10 in, 1 out]
  n5 = for {
    tunnel: w52 -> [w77] mode=indexing
    shift-right: [w69] -> w51
    shift-left: w56 -> [w78]
    tunnel: w49 -> [w75]
    n6 = property class="Ctl"(reference=w77, error in=w78) -> (reference out=w71:refnum<vi>, error out=w70:errorcluster, "Label.Text"=w76:string)
    n7 = Search 1D Array(1D array=w75, element=w76) -> (index of element=w74:i32)  [unwired: 1 in]
    n8 = Greater Or Equal?(x=w74, y=0) -> (x >= y?=w72:bool)
    n9 = case shown="True" w72 {
      tunnel: w71 -> [_ w89]
      tunnel: w70 -> [w79 w88]
      tunnel: [w79 w82] -> w69
      frame False {
      }
      frame True {
        w85 = refnum<vi> refnum  # String
        n10 = property class="Ctl"(reference=w89, error in=w88, "Visible"=TRUE, "Value"="0") -> (reference out=w87:refnum<vi>, error out=w86:errorcluster)
        n11 = To More Specific Class(target class=w85, reference=w87, error in=w86) -> (specific class reference=w84:refnum<vi>, error out=w83:errorcluster)
        n12 = property class="Str"(reference=w84, error in=w83, "Text.Justify"=enum16{"Left", "Center", "Right"}."Right" ("Text.Justification")) -> (error out=w82:errorcluster)  [unwired: 1 out]
      }
    }
  }
  n13 = control-ref of="FA Data And Events"() -> (w3:refnum<vi>)
  n14 = call "FA Data Type List.vi"("Clust Refnum"=w3, "ControlNameTypes"=enum16{"ALL", "Arrays", "SingleValues"}."ALL") -> ("Data Type List"=w18:string[], "error out"=w17:errorcluster)  [unwired: 1 out]
  n15 = control-ref of="Data Type"() -> (w63:refnum<vi>)
  n16 = property class="CmbBox"(reference=w63, error in=w17, "Strings[]"=w18, "TipStrip"="" ("Tip Strip")) -> (error out=w11:errorcluster)  [unwired: 1 out]
  n17 = call "GetM1M3SupportEvents.vi"("error in (no error)"=w11, "Model in"="Model in") -> ("error out"=w44:errorcluster, "M1M3 Support Events out"=w66:refnum<class "M1M3 Support Events.lvclass">)  [unwired: 7 in, 1 out]
  n18 = call "Get M1M3 Support Events.vi"("M1M3 Support Events in"=w66) -> ("M1M3 Support Events"=w67:T32)  [unwired: 9 in, 1 out]
  n19 = for {
    tunnel: w52 -> [w98] mode=indexing
    shift-right: [w94] -> w15
    shift-left: variant -> [w97]
    shift-right: [w91] -> w61
    shift-left: w51 -> [w93]
    n20 = property class="Ctl"(reference=w98, error in=w93) -> (reference out=w95:refnum<vi>, error out=w92:errorcluster, "Label.Text"=w96:string)
    n21 = Set Variant Attribute(Variant=w97, name=w96, value=w95, error in=w92) -> (Variant out=w94:variant, error out=w91:errorcluster)  [unwired: 1 out]
  }
  n22 = Unbundle By Name(w67) -> ("Detailed State Event"=w65:refnum<user-event>, "FA Data"=w64:refnum<user-event>, "FA Info Event"=w48:refnum<user-event>, "FA Force Warning Event"=w47:refnum<user-event>, "FA Warning Event"=w45:refnum<user-event>, "FA State Event"=w46:refnum<user-event>, "Applied AberrationForces Event"=w42:refnum<user-event>, "Applied Acceleration Forcces Event"=w41:refnum<user-event>, "Applied Azimuth Forces Event"=w40:refnum<user-event>, "Applied Active Optic Forces Event"=w39:refnum<user-event>, "Applied Balance Forces Event"=w38:refnum<user-event>, "Applied Cylinder Forces Event"=w37:refnum<user-event>, "Applied Elevation Forces Event"=w36:refnum<user-event>, "Applied Forces Event"=w35:refnum<user-event>, "Applied Offset Forces Event"=w34:refnum<user-event>, "Applied Static Forces Event"=w33:refnum<user-event>, "Applied Thermal Forces Event"=w32:refnum<user-event>, "Applied Velocity Forces Event"=w31:refnum<user-event>, "Rejected Aberration Force Event"=w30:refnum<user-event>, "Rejected Acceleration Forces Event"=w29:refnum<user-event>, "Rejected Active Optic Forces Event"=w28:refnum<user-event>, "Rejected Azimuth Forces Event"=w27:refnum<user-event>, "Rejected Balance Forces Event"=w26:refnum<user-event>, "Rejected Cylinder Forces Event"=w25:refnum<user-event>, "Rejected Elevation Forces Event"=w24:refnum<user-event>, "Rejected Forces Event"=w23:refnum<user-event>, "Rejected Offset Forces Event"=w22:refnum<user-event>, "Rejected Static Forces Event"=w21:refnum<user-event>, "Rejected Thermal Forces Event"=w20:refnum<user-event>, "Rejected Velocity Forces Event"=w19:refnum<user-event>, "Force Setpoint Warning Event"=w4:refnum<user-event>)
  n23 = register-events(error in=w44, w65, w64, w48, w47, w45, w46, w42, w41, w40, w39, w38, w37, w36, w35, w34, w33, w32, w31, w30, w29, w28, w27, w26, w25, w24, w23, w22, w21, w20, w19, w4) -> (reference out=w9:refnum<event-registration>, error out=w7:errorcluster)  [unwired: 1 in]
  n24 = Close Reference(reference=w50, error in (no error)=w61) -> (error out=w10:errorcluster)
  n25 = flat-sequence {
    tunnel: w9 -> [w101]
    tunnel: [w101] -> w8
    tunnel: w7 -> [w100]
    tunnel: [w100] -> w6
    frame #0 {
      n26 = local write "stop"(FALSE ("stop")) -> ()
    }
  }
  n27 = call "FA Number Array.vi"() -> ("FA Number Array"=w2:i32[])  [unwired: 10 in, 1 out]
  n28 = Merge Errors(w6, w10) -> (w1:errorcluster)
  n29 = while {
    tunnel: w15 -> [w112]
    shift-right: [w111] -> w14
    shift-left: w1 -> [w103]
    tunnel: [w110] -> w13
    tunnel: w2 -> [w108]
    stop <- w109 stop-if-true
    # "Reg Ex. to match bracket with number inside.  If no match, send empty string.\nThis allows us to determine wether to use the FA Controls or the Single Value."
    # "Determine which set of data the user has chosen to view and retrieve that set of data from the clusters."
    n30 = local read "stop"() -> (w109:bool)
    n31 = Match Pattern(string="Data Type", regular expression="\\-") -> (before substring=w107:string, after substring=w116:string)  [unwired: 1 in, 2 out]
    n32 = control-ref of="FA Data And Events"() -> (w102:refnum<vi>)
    n33 = Match Pattern(string=w116, regular expression="\\[[0-9]+\\]$") -> (match substring=w117:string)  [unwired: 1 in, 3 out]
    n34 = call "Get FA Data.vi"("Clust Refnum"=w102, "FA Chosen Data Type"=w107) -> ("error out"=w105:errorcluster, "ControlRefNums"=w106:refnum<vi>[])  [unwired: 8 in]
    n35 = Merge Errors(w105, w103) -> (w104:errorcluster)
    n36 = case shown="Default" w117 {
      tunnel: w104 -> [w131 w201]
      tunnel: w106 -> [w132 w200]
      tunnel: w112 -> [w130 w199]
      tunnel: [w130 w198] -> w110
      tunnel: [w128 w197] -> w111
      tunnel: w117 -> [_ w184]
      tunnel: w116 -> [w133 w195]
      tunnel: w107 -> [w118 w188]
      tunnel: w108 -> [_ w183]
      frame "" {
        # "I chose not to clear out the other controls incase someone wants to compare the values in the FA controls with the \nSingle Value control.   The Single Value wiill hightlight blue when a new value is entered so that the user will\nmore likely see the result.   The Single Value control will be empty with a gray background when data for the FA \nControls is selected."
        n37 = Concatenate Strings("m1m3_" ("string"), w118) -> (w120:string)
        n38 = property on="SingleValue" class="Str"("TipStrip"=w120) -> ()  [unwired: 2 in, 2 out]
        n39 = for {
          tunnel: w133 -> [w145]
          tunnel: w132 -> [w144] mode=indexing
          shift-right: [w136] -> w129
          shift-left: w131 -> [w143]
          shift-right: [w142] -> w122
          shift-left: "" ("StringForm") -> [w134]
          # "If a single value is selected by the user, we display it in the single value entry field."
          n40 = property class="Ctl"(reference=w144, error in=w143) -> (reference out=w148:refnum<vi>, error out=w149:errorcluster, "Label.Text"=w139:string)
          n41 = Equal?(x=w145, y=w139) -> (x = y?=w147:bool)
          n42 = property class="Ctl"(reference=w148, error in=w149) -> (reference out=w135:refnum<vi>, error out=w146:errorcluster, "Value"=w140:variant)
          n43 = Equal?(x=w139, y="timestamp") -> (x = y?=w138:bool)
          n44 = case shown="True" w138 {
            tunnel: w140 -> [_ w153]
            frame False {
            }
            frame True {
              n45 = Variant To Data(type=0.0, Variant=w153) -> (data=w151:dbl)  [unwired: 1 in, 1 out]
              n46 = call "Get Timestamp Cushion.vi"("DoubleTimestampRepresentation"=w151) -> ("TimestampCushion"=w154:dbl)  [unwired: 10 in]
              n47 = To Time Stamp(1:w154) -> (0:w150:timestamp)
              n48 = local write "Timestamp of Data being shown"(w150) -> ()
            }
          }
          n49 = case shown="True" w147 {
            tunnel: w140 -> [_ w159]
            tunnel: w146 -> [w156 w161]
            tunnel: [w156 w162] -> w137
            tunnel: [w155 w157] -> w142
            tunnel: w134 -> [w155 _]
            frame False {
            }
            frame True {
              n50 = call <vilib>:"Get Type Information.vi"("error in (no error)"=w161, "Variant"=w159) -> ("error out"=w160:errorcluster, "Type"=w158:T33)  [unwired: 5 in, 3 out]
              n51 = case shown="Default" w158 {
                tunnel: w159 -> [w169 w175 w182]
                tunnel: w160 -> [w168 w174 w181]
                tunnel: [w167 w173 w179] -> w162
                tunnel: [w163 w170 w176] -> w157
                frame "I16" {
                  n52 = Variant To Data(error in=w168, type=i16 0, Variant=w169) -> (data=w166:i16, error out=w167:errorcluster)
                  n53 = Format Into String(format string="%d", w166) -> (resulting string=w163:string)  [unwired: 2 in, 1 out]
                }
                frame "Boolean" {
                  n54 = Variant To Data(error in=w174, type=TRUE, Variant=w175) -> (data=w172:bool, error out=w173:errorcluster)
                  n55 = call "Boolean to String.vi"("BooleanValue"=w172) -> ("StringForm"=w170:string)  [unwired: 1 out]
                }
                frame Default {
                  n56 = Variant To Data(error in=w181, type=sgl 0.0, Variant=w182) -> (data=w180:sgl, error out=w179:errorcluster)
                  n57 = Format Into String(format string="%f", w180) -> (resulting string=w176:string)  [unwired: 2 in, 1 out]
                }
              }
            }
          }
          n58 = Close Reference(reference=w135, error in (no error)=w137) -> (error out=w136:errorcluster)
        }
        "SingleValue" <- w122
        n59 = Equal?(x=w122, y="True") -> (x = y?=w125:bool)
        n60 = Select(t=u32 15663118, s=w125, f=u32 9567230) -> (s? t:f=w123:u32)
        n61 = property on="SingleValue" class="Str"(error in=w129, "Text.BGColor"=w123) -> (error out=w128:errorcluster)  [unwired: 1 in, 1 out]
      }
      frame Default {
        w186 = ""
        n62 = for {
          tunnel: w195 -> [w213]
          tunnel: w200 -> [w212] mode=indexing
          shift-right: [w205] -> w190
          shift-left: string[] [] -> [w206]
          shift-right: [w203] -> w194
          shift-left: w201 -> [w211]
          n63 = property class="Ctl"(reference=w212, error in=w211) -> (reference out=w216:refnum<vi>, error out=w217:errorcluster, "Label.Text"=w209:string)
          n64 = Equal?(x=w213, y=w209) -> (x = y?=w215:bool)
          n65 = property class="Ctl"(reference=w216, error in=w217) -> (reference out=w202:refnum<vi>, error out=w214:errorcluster, "Value"=w207:variant)
          n66 = Equal?(x=w209, y="Timestamp") -> (x = y?=w210:bool)
          n67 = case shown="True" w210 {
            tunnel: w207 -> [_ w220]
            frame False {
            }
            frame True {
              n68 = Variant To Data(type=0.0, Variant=w220) -> (data=w218:dbl)  [unwired: 1 in, 1 out]
              n69 = call "Get Timestamp Cushion.vi"("DoubleTimestampRepresentation"=w218) -> ("TimestampCushion"=w222:dbl)  [unwired: 10 in]
              n70 = To Time Stamp(1:w222) -> (0:→"Timestamp of Data being shown":timestamp)
            }
          }
          n71 = case shown="True" w215 {
            tunnel: w207 -> [_ w227]
            tunnel: w214 -> [w224 w228]
            tunnel: [w224 w225] -> w204
            tunnel: w206 -> [w223 _]
            tunnel: [w223 w226] -> w205
            frame False {
            }
            frame True {
              n72 = call "Variant Array to String Array.vi"("error in (no error)"=w228, "Variant"=w227) -> ("error out"=w225:errorcluster, "String Array"=w226:string[])  [unwired: 8 in]
            }
          }
          n73 = Close Reference(reference=w202, error in (no error)=w204) -> (error out=w203:errorcluster)
        }
        n74 = call "Data Type to FA Array.vi"("Data Type"=w184) -> ("On/Off Array"=w185:bool[])  [unwired: 10 in]
        n75 = property on="SingleValue" class="Str"(error in=w194, "Text.BGColor"=u32 16777238, "Value"=w186, "TipStrip"=w186) -> (error out=w193:errorcluster)  [unwired: 1 in, 1 out]
        n76 = Concatenate Strings("m1m3_" ("string"), w188) -> (w189:string)
        n77 = for {
          tunnel: w183 -> [w248] mode=indexing
          tunnel: w185 -> [w233] mode=indexing
          shift-right: [w237] -> w197
          shift-left: w193 -> [w236]
          tunnel: w199 -> [w235]
          tunnel: [w234] -> w198
          shift-right: [w231] -> _
          shift-left: 0 -> [w232]
          tunnel: w190 -> [w230]
          tunnel: w189 -> [w229]
          # "Go through the FA numbers and use them to \nretrieve the appropriate control reference on the\npanel.  Then determine that control's visibility and\nload the data into said control."
          n78 = Format Into String(format string="%d", w248) -> (resulting string=w246:string)  [unwired: 2 in, 1 out]
          n79 = Get Variant Attribute(Variant=w235, name=w246, default value (empty Variant)=variant ("default value (empty variant)"), error in=w236) -> (duplicate Variant=w234:variant, value=w243:variant, error out=w241:errorcluster)  [unwired: 1 out]
          n80 = Variant To Data(error in=w241, type=refnum<vi> refnum ("reference out"), Variant=w243) -> (data=w240:refnum<vi>, error out=w239:errorcluster)
          n81 = property class="Ctl"(reference=w240, error in=w239, "Visible"=w233) -> (reference out=w242:refnum<vi>, error out=w238:errorcluster)
          n82 = case shown="True" w233 {
            tunnel: w230 -> [_ w269]
            tunnel: w242 -> [w250 w271]
            tunnel: w238 -> [w252 w270]
            tunnel: [w251 w255] -> w237
            tunnel: w232 -> [w253 w262]
            tunnel: [w253 w268] -> w231
            tunnel: w229 -> [_ w254]
            frame False {
              n83 = property class="Ctl"(reference=w250, error in=w252, "Value"="0.000") -> (error out=w251:errorcluster)  [unwired: 1 out]
            }
            frame True {
              w265 = refnum<vi> refnum  # String
              n84 = Index Array(array=w269, index=w262) -> (element=w261:string)
              n85 = Increment(x=w262) -> (x+1=w268:i32)
              n86 = Equal?(x=w261, y="True") -> (x = y?=w259:bool)
              n87 = property class="Ctl"(reference=w271, error in=w270, "Value"=w261, "TipStrip"=w254) -> (reference out=w266:refnum<vi>, error out=w267:errorcluster)
              n88 = To More Specific Class(target class=w265, reference=w266, error in=w267) -> (specific class reference=w264:refnum<vi>, error out=w263:errorcluster)
              n89 = Select(t=u32 15663118, s=w259, f=u32 16777238) -> (s? t:f=w256:u32)
              n90 = property class="Str"(reference=w264, error in=w263, "Text.BGColor"=w256) -> (error out=w255:errorcluster)  [unwired: 1 out]
            }
          }
        }
      }
    }
  }
  n91 = while {
    tunnel: w8 -> [w276]
    tunnel: [w275] -> w58
    shift-right: [w273] -> _
    shift-left: "FA Data And Events" -> [w274]
    stop <- w272 stop-if-true
    n92 = event shown="[29] <Force Setpoint Warning Event>: User Event" {
      selector: w276 -> [_ _ _ _ _ _ _ _ _ _ _ _ _ _ _ _ _ _ _ _ _ _ _ _ _ _ _ _ _ _]
      dyn-events: [_ _ _ _ _ _ _ _ _ _ _ _ _ _ _ _ _ _ _ _ _ _ _ _ _ _ _ _ _ _] -> w275
      timeout: _ -> [_ _ _ _ _ _ _ _ _ _ _ _ _ _ _ _ _ _ _ _ _ _ _ _ _ _ _ _ _ _]
      tunnel: [w280 FALSE _ _ _ _ _ _ _ _ _ _ _ _ _ _ _ _ _ _ _ _ _ _ _ _ _ _ _ _] -> w272
      tunnel: w274 -> [w279 w290 w301 w368 w387 w430 w445 w454 w469 w484 w493 w508 w515 w530 w545 w560 w574 w590 w605 w614 w629 w638 w653 w668 w675 w690 w705 w720 w735 w787]
      tunnel: [w279 w288 w300 w366 w386 w429 w443 w452 w467 w482 w491 w506 w513 w528 w543 w558 w573 w588 w603 w612 w627 w636 w651 w666 w673 w688 w703 w718 w733 w785] -> w273
      event User Event {
        n93 = event-data() -> ("DetailedState"=w278:T34)  [unwired: 1 in]
        n94 = Equal?(x=w278, y=T34."DetailedState_DetailedStates_OfflineState") -> (x = y?=w280:bool)
      }
      event User Event {
        n95 = event-data() -> ("Timestamp"=w292:dbl, "PrimaryCylinderForce[156]"=w297:sgl[], "SecondaryCylinderForce[112]"=w296:sgl[], "XForce[12]"=w295:sgl[], "YForce[100]"=w294:sgl[], "ZForce[156]"=w293:sgl[], "Fx"=w287:sgl, "Fy"=w286:sgl, "Fz"=w285:sgl, "Mx"=w284:sgl, "My"=w283:sgl, "Mz"=w282:sgl, "ForceMagnitude"=w281:sgl)  [unwired: 1 in, 4 out]
        n96 = Unbundle By Name(w290) -> ("ForceActuatorData"=w291:T2)
        n97 = Bundle By Name(cluster=w291, "Timestamp"=w292, "PrimaryCylinderForce[156]"=w297, "SecondaryCylinderForce[112]"=w296, "XForce[12]"=w295, "YForce[100]"=w294, "ZForce[156]"=w293, "Fx"=w287, "Fy"=w286, "Fz"=w285, "Mx"=w284, "My"=w283, "Mz"=w282, "ForceMagnitude"=w281) -> (w289:T2)
        n98 = Bundle By Name(cluster=w290, "ForceActuatorData"=w289) -> (w288:T1)
      }
      event User Event {
        n99 = event-data() -> ("Timestamp"=w303:dbl, "AnyWarning"=w365:bool, "AnyMajorFault"=w364:bool, "MajorFault[156]"=w363:bool[], "AnyMinorFault"=w362:bool, "MinorFault[156]"=w361:bool[], "AnyFaultOverride"=w360:bool, "FaultOverride[156]"=w359:bool[], "AnyMainCalibrationError"=w358:bool, "MainCalibrationError[156]"=w357:bool[], "AnyBackupCalibrationError"=w356:bool, "BackupCalibrationError[156]"=w355:bool[], "AnyMezzanineError"=w354:bool, "MezzanineError[156]"=w353:bool[], "AnyMezzanineBootloaderActive"=w352:bool, "MezzanineBootloaderActive[156]"=w351:bool[], "AnyUniqueIdCRCError"=w350:bool, "UniqueIdCRCError[156]"=w349:bool[], "AnyApplicationTypeMismatch"=w348:bool, "ApplicationTypeMismatch[156]"=w347:bool[], "AnyApplicationMissing"=w346:bool, "ApplicationMissing[156]"=w345:bool[], "AnyApplicationCRCMismatch"=w344:bool, "ApplicationCRCMismatch[156]"=w343:bool[], "AnyOneWireMissing"=w342:bool, "OneWireMissing[156]"=w341:bool[], "AnyOneWire1Mismatch"=w340:bool, "OneWire1Mismatch[156]"=w339:bool[], "AnyOneWire2Mismatch"=w338:bool, "OneWire2Mismatch[156]"=w337:bool[], "AnyWatchdogReset"=w336:bool, "WatchdogReset[156]"=w335:bool[], "AnyBrownOut"=w334:bool, "BrownOut[156]"=w333:bool[], "AnyEventTrapReset"=w332:bool, "EventTrapReset[156]"=w331:bool[], "AnySSRPowerFault"=w330:bool, "SSRPowerFault[156]"=w329:bool[], "AnyAuxPowerFault"=w328:bool, "AuxPowerFault[156]"=w327:bool[], "AnyMezzaninePowerFault"=w326:bool, "MezzaninePowerFault[156]"=w325:bool[], "AnyMezzanineCurrentAmp1Fault"=w324:bool, "MezzanineCurrentAmp1Fault[156]"=w323:bool[], "AnyMezzanineCurrentAmp2Fault"=w322:bool, "MezzanineCurrentAmp2Fault[156]"=w321:bool[], "AnyMezzanineUniqueIdCRCError"=w320:bool, "MezzanineUniqueIdCRCError[156]"=w319:bool[], "AnyMezzanineMainCalibrationError"=w318:bool, "MezzanineMainCalibrationError[156]"=w317:bool[], "AnyMezzanineBackupCalibrationError"=w316:bool, "MezzanineBackupCalibrationError[156]"=w315:bool[], "AnyMezzanineEventTrapReset"=w314:bool, "MezzanineEventTrapReset[156]"=w313:bool[], "AnyMezzanineApplicationMissing"=w312:bool, "MezzanineApplicationMissing[156]"=w311:bool[], "AnyMezzanineApplicationCRCMismatch"=w310:bool, "MezzanineApplicationCRCMismatch[156]"=w309:bool[], "AnyILCFault"=w308:bool, "ILCFault[156]"=w307:bool[], "AnyBroadcastCounterWarning"=w306:bool, "BroadcastCounterWarning[156]"=w305:bool[], "priority"=w304:i32)  [unwired: 1 in, 4 out]
        n100 = Unbundle By Name(w301) -> ("logevent_ForceActuatorWarning"=w302:T6)
        n101 = Bundle By Name(cluster=w302, "Timestamp"=w303, "AnyWarning"=w365, "AnyMajorFault"=w364, "MajorFault[156]"=w363, "AnyMinorFault"=w362, "MinorFault[156]"=w361, "AnyFaultOverride"=w360, "FaultOverride[156]"=w359, "AnyMainCalibrationError"=w358, "MainCalibrationError[156]"=w357, "AnyBackupCalibrationError"=w356, "BackupCalibrationError[156]"=w355, "AnyMezzanineError"=w354, "MezzanineError[156]"=w353, "AnyMezzanineBootloaderActive"=w352, "MezzanineBootloaderActive[156]"=w351, "AnyUniqueIdCRCError"=w350, "UniqueIdCRCError[156]"=w349, "AnyApplicationTypeMismatch"=w348, "ApplicationTypeMismatch[156]"=w347, "AnyApplicationMissing"=w346, "ApplicationMissing[156]"=w345, "AnyApplicationCRCMismatch"=w344, "ApplicationCRCMismatch[156]"=w343, "AnyOneWireMissing"=w342, "OneWireMissing[156]"=w341, "AnyOneWire1Mismatch"=w340, "OneWire1Mismatch[156]"=w339, "AnyOneWire2Mismatch"=w338, "OneWire2Mismatch[156]"=w337, "AnyWatchdogReset"=w336, "WatchdogReset[156]"=w335, "AnyBrownOut"=w334, "BrownOut[156]"=w333, "AnyEventTrapReset"=w332, "EventTrapReset[156]"=w331, "AnySSRPowerFault"=w330, "SSRPowerFault[156]"=w329, "AnyAuxPowerFault"=w328, "AuxPowerFault[156]"=w327, "AnyMezzaninePowerFault"=w326, "MezzaninePowerFault[156]"=w325, "AnyMezzanineCurrentAmp1Fault"=w324, "MezzanineCurrentAmp1Fault[156]"=w323, "AnyMezzanineCurrentAmp2Fault"=w322, "MezzanineCurrentAmp2Fault[156]"=w321, "AnyMezzanineUniqueIdCRCError"=w320, "MezzanineUniqueIdCRCError[156]"=w319, "AnyMezzanineMainCalibrationError"=w318, "MezzanineMainCalibrationError[156]"=w317, "AnyMezzanineBackupCalibrationError"=w316, "MezzanineBackupCalibrationError[156]"=w315, "AnyMezzanineEventTrapReset"=w314, "MezzanineEventTrapReset[156]"=w313, "AnyMezzanineApplicationMissing"=w312, "MezzanineApplicationMissing[156]"=w311, "AnyMezzanineApplicationCRCMismatch"=w310, "MezzanineApplicationCRCMismatch[156]"=w309, "AnyILCFault"=w308, "ILCFault[156]"=w307, "AnyBroadcastCounterWarning"=w306, "BroadcastCounterWarning[156]"=w305, "priority"=w304) -> (w299:T6)
        n102 = Bundle By Name(cluster=w301, "logevent_ForceActuatorWarning"=w299) -> (w300:T1)
      }
      event User Event {
        n103 = event-data() -> ("Timestamp"=w370:dbl, "ILCState[156]"=w384:i16[], "SlewFlag"=w383:bool, "StaticForcesApplied"=w382:bool, "ElevationForcesApplied"=w381:bool, "AzimuthForcesApplied"=w380:bool, "ThermalForcesApplied"=w379:bool, "OffsetForcesApplied"=w378:bool, "AccelerationForcesApplied"=w377:bool, "VelocityForcesApplied"=w376:bool, "ActiveOpticForcesApplied"=w375:bool, "AberrationForcesApplied"=w374:bool, "BalanceForcesApplied"=w373:bool, "SupportPercentage"=w372:sgl, "priority"=w371:i32)  [unwired: 1 in, 4 out]
        n104 = Unbundle By Name(w368) -> ("logevent_ForceActuatorState"=w369:T5)
        n105 = Bundle By Name(cluster=w369, "Timestamp"=w370, "ILCState[156]"=w384, "SlewFlag"=w383, "StaticForcesApplied"=w382, "ElevationForcesApplied"=w381, "AzimuthForcesApplied"=w380, "ThermalForcesApplied"=w379, "OffsetForcesApplied"=w378, "AccelerationForcesApplied"=w377, "VelocityForcesApplied"=w376, "ActiveOpticForcesApplied"=w375, "AberrationForcesApplied"=w374, "BalanceForcesApplied"=w373, "SupportPercentage"=w372, "priority"=w371) -> (w367:T5)
        n106 = Bundle By Name(cluster=w368, "logevent_ForceActuatorState"=w367) -> (w366:T1)
      }
      event User Event {
        n107 = event-data() -> ("Timestamp"=w389:dbl, "ReferenceId[156]"=w427:i16[], "XDataReferenceId[12]"=w426:i16[], "YDataReferenceId[100]"=w425:i16[], "ZDataReferenceId[156]"=w424:i16[], "ActuatorType[156]"=w423:i16[], "ActuatorOrientation[156]"=w422:i16[], "ModbusSubnet[156]"=w421:i16[], "ModbusAddress[156]"=w420:i16[], "XPosition[156]"=w419:sgl[], "YPosition[156]"=w418:sgl[], "ZPosition[156]"=w417:sgl[], "ILCUniqueId[156]"=w416:i64[], "ILCApplicationType[156]"=w415:i16[], "NetworkNodeType[156]"=w414:i16[], "ILCSelectedOptions[156]"=w413:i16[], "NetworkNodeOptions[156]"=w412:i16[], "MajorRevision[156]"=w411:i16[], "MinorRevision[156]"=w410:i16[], "ADCScanRate[156]"=w409:i16[], "MainPrimaryCylinderCoefficient[156]"=w408:sgl[], "MainSecondaryCylinderCoefficient[156]"=w407:sgl[], "MainPrimaryCylinderLoadCellOffset[156]"=w406:sgl[], "MainSecondaryCylinderLoadCellOffset[156]"=w405:sgl[], "MainPrimaryCylinderLoadCellSensitivity[156]"=w404:sgl[], "MainSecondaryCylinderLoadCellSensitivity[156]"=w403:sgl[], "BackupPrimaryCylinderCoefficient[156]"=w402:sgl[], "BackupSecondaryCylinderCoefficient[156]"=w401:sgl[], "BackupPrimaryCylinderLoadCellOffset[156]"=w400:sgl[], "BackupSecondaryCylinderLoadCellOffset[156]"=w399:sgl[], "BackupPrimaryCylinderLoadCellSensitivity[156]"=w398:sgl[], "BackupSecondaryCylinderLoadCellSensitivity[156]"=w397:sgl[], "MezzaninePrimaryCylinderGain[156]"=w396:sgl[], "MezzanineSecondaryCylinderGain[156]"=w395:sgl[], "MezzanineUniqueId[156]"=w394:i64[], "MezzanineFirmwareType[156]"=w393:i16[], "MezzanineMajorRevision[156]"=w392:i16[], "MezzanineMinorRevision[156]"=w391:i16[], "priority"=w390:i32)  [unwired: 1 in, 4 out]
        n108 = Unbundle By Name(w387) -> ("logevent_ForceActuatorInfo"=w388:T4)
        n109 = Bundle By Name(cluster=w388, "Timestamp"=w389, "ReferenceId[156]"=w427, "XDataReferenceId[12]"=w426, "YDataReferenceId[100]"=w425, "ZDataReferenceId[156]"=w424, "ActuatorType[156]"=w423, "ActuatorOrientation[156]"=w422, "ModbusSubnet[156]"=w421, "ModbusAddress[156]"=w420, "XPosition[156]"=w419, "YPosition[156]"=w418, "ZPosition[156]"=w417, "ILCUniqueId[156]"=w416, "ILCApplicationType[156]"=w415, "NetworkNodeType[156]"=w414, "ILCSelectedOptions[156]"=w413, "NetworkNodeOptions[156]"=w412, "MajorRevision[156]"=w411, "MinorRevision[156]"=w410, "ADCScanRate[156]"=w409, "MainPrimaryCylinderCoefficient[156]"=w408, "MainSecondaryCylinderCoefficient[156]"=w407, "MainPrimaryCylinderLoadCellOffset[156]"=w406, "MainSecondaryCylinderLoadCellOffset[156]"=w405, "MainPrimaryCylinderLoadCellSensitivity[156]"=w404, "MainSecondaryCylinderLoadCellSensitivity[156]"=w403, "BackupPrimaryCylinderCoefficient[156]"=w402, "BackupSecondaryCylinderCoefficient[156]"=w401, "BackupPrimaryCylinderLoadCellOffset[156]"=w400, "BackupSecondaryCylinderLoadCellOffset[156]"=w399, "BackupPrimaryCylinderLoadCellSensitivity[156]"=w398, "BackupSecondaryCylinderLoadCellSensitivity[156]"=w397, "MezzaninePrimaryCylinderGain[156]"=w396, "MezzanineSecondaryCylinderGain[156]"=w395, "MezzanineUniqueId[156]"=w394, "MezzanineFirmwareType[156]"=w393, "MezzanineMajorRevision[156]"=w392, "MezzanineMinorRevision[156]"=w391, "priority"=w390) -> (w385:T4)
        n110 = Bundle By Name(cluster=w387, "logevent_ForceActuatorInfo"=w385) -> (w386:T1)
      }
      event User Event {
        n111 = event-data() -> ("Timestamp"=w432:dbl, "AnyWarning"=w442:bool, "AnyPrimaryAxisMeasuredForceWarning"=w441:bool, "PrimaryAxisMeasuredForceWarning[156]"=w440:bool[], "AnySecondaryAxisMeasuredForceWarning"=w439:bool, "SecondaryAxisMeasuredForceWarning[156]"=w438:bool[], "AnyPrimaryAxisFollowingErrorWarning"=w437:bool, "PrimaryAxisFollowingErrorWarning[156]"=w436:bool[], "AnySecondaryAxisFollowingErrorWarning"=w435:bool, "SecondaryAxisFollowingErrorWarning[156]"=w434:bool[], "priority"=w433:i32)  [unwired: 1 in, 4 out]
        n112 = Unbundle By Name(w430) -> ("logevent_ForceActuatorForceWarning"=w431:T3)
        n113 = Bundle By Name(cluster=w431, "Timestamp"=w432, "AnyWarning"=w442, "AnyPrimaryAxisMeasuredForceWarning"=w441, "PrimaryAxisMeasuredForceWarning[156]"=w440, "AnySecondaryAxisMeasuredForceWarning"=w439, "SecondaryAxisMeasuredForceWarning[156]"=w438, "AnyPrimaryAxisFollowingErrorWarning"=w437, "PrimaryAxisFollowingErrorWarning[156]"=w436, "AnySecondaryAxisFollowingErrorWarning"=w435, "SecondaryAxisFollowingErrorWarning[156]"=w434, "priority"=w433) -> (w428:T3)
        n114 = Bundle By Name(cluster=w430, "logevent_ForceActuatorForceWarning"=w428) -> (w429:T1)
      }
      event User Event {
        n115 = event-data() -> ("Timestamp"=w450:dbl, "ZForces[156]"=w449:sgl[], "Fz"=w448:sgl, "Mx"=w447:sgl, "My"=w446:sgl)  [unwired: 1 in, 4 out]
        n116 = Unbundle By Name(w445) -> ("logevent_AppliedAberrationForces"=w451:T7)
        n117 = Bundle By Name(cluster=w451, "Timestamp"=w450, "ZForces[156]"=w449, "Fz"=w448, "Mx"=w447, "My"=w446) -> (w444:T7)
        n118 = Bundle By Name(cluster=w445, "logevent_AppliedAberrationForces"=w444) -> (w443:T1)
      }
      event User Event {
        n119 = event-data() -> ("Timestamp"=w465:dbl, "XForces[12]"=w464:sgl[], "YForces[100]"=w463:sgl[], "ZForces[156]"=w462:sgl[], "Fx"=w461:sgl, "Fy"=w460:sgl, "Fz"=w459:sgl, "Mx"=w458:sgl, "My"=w457:sgl, "Mz"=w456:sgl, "ForceMagnitude"=w455:sgl)  [unwired: 1 in, 5 out]
        n120 = Unbundle By Name(w454) -> ("logevent_AppliedAccelerationForces"=w466:T8)
        n121 = Bundle By Name(cluster=w466, "Timestamp"=w465, "XForces[12]"=w464, "YForces[100]"=w463, "ZForces[156]"=w462, "Fx"=w461, "Fy"=w460, "Fz"=w459, "Mx"=w458, "My"=w457, "Mz"=w456, "ForceMagnitude"=w455) -> (w453:T8)
        n122 = Bundle By Name(cluster=w454, "logevent_AppliedAccelerationForces"=w453) -> (w452:T1)
      }
      event User Event {
        n123 = event-data() -> ("Timestamp"=w480:dbl, "XForces[12]"=w479:sgl[], "YForces[100]"=w478:sgl[], "ZForces[156]"=w477:sgl[], "Fx"=w476:sgl, "Fy"=w475:sgl, "Fz"=w474:sgl, "Mx"=w473:sgl, "My"=w472:sgl, "Mz"=w471:sgl, "ForceMagnitude"=w470:sgl)  [unwired: 1 in, 4 out]
        n124 = Unbundle By Name(w469) -> ("logevent_AppliedAzimuthForces"=w481:T10)
        n125 = Bundle By Name(cluster=w481, "Timestamp"=w480, "XForces[12]"=w479, "YForces[100]"=w478, "ZForces[156]"=w477, "Fx"=w476, "Fy"=w475, "Fz"=w474, "Mx"=w473, "My"=w472, "Mz"=w471, "ForceMagnitude"=w470) -> (w468:T10)
        n126 = Bundle By Name(cluster=w469, "logevent_AppliedAzimuthForces"=w468) -> (w467:T1)
      }
      event User Event {
        n127 = event-data() -> ("Timestamp"=w489:dbl, "ZForces[156]"=w488:sgl[], "Fz"=w487:sgl, "Mx"=w486:sgl, "My"=w485:sgl)  [unwired: 1 in, 4 out]
        n128 = Unbundle By Name(w484) -> ("logevent_AppliedActiveOpticForces"=w490:T9)
        n129 = Bundle By Name(cluster=w490, "Timestamp"=w489, "ZForces[156]"=w488, "Fz"=w487, "Mx"=w486, "My"=w485) -> (w483:T9)
        n130 = Bundle By Name(cluster=w484, "logevent_AppliedActiveOpticForces"=w483) -> (w482:T1)
      }
      event User Event {
        n131 = event-data() -> ("Timestamp"=w504:dbl, "XForces[12]"=w503:sgl[], "YForces[100]"=w502:sgl[], "ZForces[156]"=w501:sgl[], "Fx"=w500:sgl, "Fy"=w499:sgl, "Fz"=w498:sgl, "Mx"=w497:sgl, "My"=w496:sgl, "Mz"=w495:sgl, "ForceMagnitude"=w494:sgl)  [unwired: 1 in, 4 out]
        n132 = Unbundle By Name(w493) -> ("logevent_AppliedBalanceForces"=w505:T11)
        n133 = Bundle By Name(cluster=w505, "Timestamp"=w504, "XForces[12]"=w503, "YForces[100]"=w502, "ZForces[156]"=w501, "Fx"=w500, "Fy"=w499, "Fz"=w498, "Mx"=w497, "My"=w496, "Mz"=w495, "ForceMagnitude"=w494) -> (w492:T11)
        n134 = Bundle By Name(cluster=w493, "logevent_AppliedBalanceForces"=w492) -> (w491:T1)
      }
      event User Event {
        n135 = event-data() -> ("Timestamp"=w511:dbl, "SecondaryCylinderForces[112]"=w510:i32[], "PrimaryCylinderForces[156]"=w509:i32[])  [unwired: 1 in, 4 out]
        n136 = Unbundle By Name(w508) -> ("logevent_AppliedCylinderForces"=w512:T12)
        n137 = Bundle By Name(cluster=w512, "Timestamp"=w511, "SecondaryCylinderForces[112]"=w510, "PrimaryCylinderForces[156]"=w509) -> (w507:T12)
        n138 = Bundle By Name(cluster=w508, "logevent_AppliedCylinderForces"=w507) -> (w506:T1)
      }
      event User Event {
        n139 = event-data() -> ("Timestamp"=w526:dbl, "XForces[12]"=w525:sgl[], "YForces[100]"=w524:sgl[], "ZForces[156]"=w523:sgl[], "Fx"=w522:sgl, "Fy"=w521:sgl, "Fz"=w520:sgl, "Mx"=w519:sgl, "My"=w518:sgl, "Mz"=w517:sgl, "ForceMagnitude"=w516:sgl)  [unwired: 1 in, 4 out]
        n140 = Unbundle By Name(w515) -> ("logevent_AppliedElevationForces"=w527:T13)
        n141 = Bundle By Name(cluster=w527, "Timestamp"=w526, "XForces[12]"=w525, "YForces[100]"=w524, "ZForces[156]"=w523, "Fx"=w522, "Fy"=w521, "Fz"=w520, "Mx"=w519, "My"=w518, "Mz"=w517, "ForceMagnitude"=w516) -> (w514:T13)
        n142 = Bundle By Name(cluster=w515, "logevent_AppliedElevationForces"=w514) -> (w513:T1)
      }
      event User Event {
        n143 = event-data() -> ("Timestamp"=w541:dbl, "XForces[12]"=w540:sgl[], "YForces[100]"=w539:sgl[], "ZForces[156]"=w538:sgl[], "Fx"=w537:sgl, "Fy"=w536:sgl, "Fz"=w535:sgl, "Mx"=w534:sgl, "My"=w533:sgl, "Mz"=w532:sgl, "ForceMagnitude"=w531:sgl)  [unwired: 1 in, 4 out]
        n144 = Unbundle By Name(w530) -> ("logevent_AppliedForces"=w542:T14)
        n145 = Bundle By Name(cluster=w542, "Timestamp"=w541, "XForces[12]"=w540, "YForces[100]"=w539, "ZForces[156]"=w538, "Fx"=w537, "Fy"=w536, "Fz"=w535, "Mx"=w534, "My"=w533, "Mz"=w532, "ForceMagnitude"=w531) -> (w529:T14)
        n146 = Bundle By Name(cluster=w530, "logevent_AppliedForces"=w529) -> (w528:T1)
      }
      event User Event {
        n147 = event-data() -> ("Timestamp"=w556:dbl, "XForces[12]"=w555:sgl[], "YForces[100]"=w554:sgl[], "ZForces[156]"=w553:sgl[], "Fx"=w552:sgl, "Fy"=w551:sgl, "Fz"=w550:sgl, "Mx"=w549:sgl, "My"=w548:sgl, "Mz"=w547:sgl, "ForceMagnitude"=w546:sgl)  [unwired: 1 in, 4 out]
        n148 = Unbundle By Name(w545) -> ("logevent_AppliedOffsetForces"=w557:T15)
        n149 = Bundle By Name(cluster=w557, "Timestamp"=w556, "XForces[12]"=w555, "YForces[100]"=w554, "ZForces[156]"=w553, "Fx"=w552, "Fy"=w551, "Fz"=w550, "Mx"=w549, "My"=w548, "Mz"=w547, "ForceMagnitude"=w546) -> (w544:T15)
        n150 = Bundle By Name(cluster=w545, "logevent_AppliedOffsetForces"=w544) -> (w543:T1)
      }
      event User Event {
        n151 = event-data() -> ("Timestamp"=w571:dbl, "XForces[12]"=w570:sgl[], "YForces[100]"=w569:sgl[], "ZForces[156]"=w568:sgl[], "Fx"=w567:sgl, "Fy"=w566:sgl, "Fz"=w565:sgl, "Mx"=w564:sgl, "My"=w563:sgl, "Mz"=w562:sgl, "ForceMagnitude"=w561:sgl)  [unwired: 1 in, 4 out]
        n152 = Unbundle By Name(w560) -> ("logevent_AppliedStaticForces"=w572:T16)
        n153 = Bundle By Name(cluster=w572, "Timestamp"=w571, "XForces[12]"=w570, "YForces[100]"=w569, "ZForces[156]"=w568, "Fx"=w567, "Fy"=w566, "Fz"=w565, "Mx"=w564, "My"=w563, "Mz"=w562, "ForceMagnitude"=w561) -> (w559:T16)
        n154 = Bundle By Name(cluster=w560, "logevent_AppliedStaticForces"=w559) -> (w558:T1)
      }
      event User Event {
        n155 = event-data() -> ("Timestamp"=w586:dbl, "XForces[12]"=w585:sgl[], "YForces[100]"=w584:sgl[], "ZForces[156]"=w583:sgl[], "Fx"=w582:sgl, "Fy"=w581:sgl, "Fz"=w580:sgl, "Mx"=w579:sgl, "My"=w578:sgl, "Mz"=w577:sgl, "ForceMagnitude"=w576:sgl)  [unwired: 1 in, 5 out]
        n156 = Unbundle By Name(w574) -> ("logevent_AppliedThermalForces"=w587:T17)
        n157 = Bundle By Name(cluster=w587, "Timestamp"=w586, "XForces[12]"=w585, "YForces[100]"=w584, "ZForces[156]"=w583, "Fx"=w582, "Fy"=w581, "Fz"=w580, "Mx"=w579, "My"=w578, "Mz"=w577, "ForceMagnitude"=w576) -> (w575:T17)
        n158 = Bundle By Name(cluster=w574, "logevent_AppliedThermalForces"=w575) -> (w573:T1)
      }
      event User Event {
        n159 = event-data() -> ("Timestamp"=w601:dbl, "XForces[12]"=w600:sgl[], "YForces[100]"=w599:sgl[], "ZForces[156]"=w598:sgl[], "Fx"=w597:sgl, "Fy"=w596:sgl, "Fz"=w595:sgl, "Mx"=w594:sgl, "My"=w593:sgl, "Mz"=w592:sgl, "ForceMagnitude"=w591:sgl)  [unwired: 1 in, 4 out]
        n160 = Unbundle By Name(w590) -> ("logevent_AppliedVelocityForces"=w602:T18)
        n161 = Bundle By Name(cluster=w602, "Timestamp"=w601, "XForces[12]"=w600, "YForces[100]"=w599, "ZForces[156]"=w598, "Fx"=w597, "Fy"=w596, "Fz"=w595, "Mx"=w594, "My"=w593, "Mz"=w592, "ForceMagnitude"=w591) -> (w589:T18)
        n162 = Bundle By Name(cluster=w590, "logevent_AppliedVelocityForces"=w589) -> (w588:T1)
      }
      event User Event {
        n163 = event-data() -> ("Timestamp"=w610:dbl, "ZForces[156]"=w609:sgl[], "Fz"=w608:sgl, "Mx"=w607:sgl, "My"=w606:sgl)  [unwired: 1 in, 4 out]
        n164 = Unbundle By Name(w605) -> ("logevent_RejectedAberrationForces"=w611:T19)
        n165 = Bundle By Name(cluster=w611, "Timestamp"=w610, "ZForces[156]"=w609, "Fz"=w608, "Mx"=w607, "My"=w606) -> (w604:T19)
        n166 = Bundle By Name(cluster=w605, "logevent_RejectedAberrationForces"=w604) -> (w603:T1)
      }
      event User Event {
        n167 = event-data() -> ("Timestamp"=w625:dbl, "XForces[12]"=w624:sgl[], "YForces[100]"=w623:sgl[], "ZForces[156]"=w622:sgl[], "Fx"=w621:sgl, "Fy"=w620:sgl, "Fz"=w619:sgl, "Mx"=w618:sgl, "My"=w617:sgl, "Mz"=w616:sgl, "ForceMagnitude"=w615:sgl)  [unwired: 1 in, 4 out]
        n168 = Unbundle By Name(w614) -> ("logevent_RejectedAccelerationForces"=w626:T20)
        n169 = Bundle By Name(cluster=w626, "Timestamp"=w625, "XForces[12]"=w624, "YForces[100]"=w623, "ZForces[156]"=w622, "Fx"=w621, "Fy"=w620, "Fz"=w619, "Mx"=w618, "My"=w617, "Mz"=w616, "ForceMagnitude"=w615) -> (w613:T20)
        n170 = Bundle By Name(cluster=w614, "logevent_RejectedAccelerationForces"=w613) -> (w612:T1)
      }
      event User Event {
        n171 = event-data() -> ("Timestamp"=w634:dbl, "ZForces[156]"=w633:sgl[], "Fz"=w632:sgl, "Mx"=w631:sgl, "My"=w630:sgl)  [unwired: 1 in, 4 out]
        n172 = Unbundle By Name(w629) -> ("logevent_RejectedActiveOpticForces"=w635:T21)
        n173 = Bundle By Name(cluster=w635, "Timestamp"=w634, "ZForces[156]"=w633, "Fz"=w632, "Mx"=w631, "My"=w630) -> (w628:T21)
        n174 = Bundle By Name(cluster=w629, "logevent_RejectedActiveOpticForces"=w628) -> (w627:T1)
      }
      event User Event {
        n175 = event-data() -> ("Timestamp"=w649:dbl, "XForces[12]"=w648:sgl[], "YForces[100]"=w647:sgl[], "ZForces[156]"=w646:sgl[], "Fx"=w645:sgl, "Fy"=w644:sgl, "Fz"=w643:sgl, "Mx"=w642:sgl, "My"=w641:sgl, "Mz"=w640:sgl, "ForceMagnitude"=w639:sgl)  [unwired: 1 in, 4 out]
        n176 = Unbundle By Name(w638) -> ("logevent_RejectedAzimuthForces"=w650:T22)
        n177 = Bundle By Name(cluster=w650, "Timestamp"=w649, "XForces[12]"=w648, "YForces[100]"=w647, "ZForces[156]"=w646, "Fx"=w645, "Fy"=w644, "Fz"=w643, "Mx"=w642, "My"=w641, "Mz"=w640, "ForceMagnitude"=w639) -> (w637:T22)
        n178 = Bundle By Name(cluster=w638, "logevent_RejectedAzimuthForces"=w637) -> (w636:T1)
      }
      event User Event {
        n179 = event-data() -> ("Timestamp"=w664:dbl, "XForces[12]"=w663:sgl[], "YForces[100]"=w662:sgl[], "ZForces[156]"=w661:sgl[], "Fx"=w660:sgl, "Fy"=w659:sgl, "Fz"=w658:sgl, "Mx"=w657:sgl, "My"=w656:sgl, "Mz"=w655:sgl, "ForceMagnitude"=w654:sgl)  [unwired: 1 in, 4 out]
        n180 = Unbundle By Name(w653) -> ("logevent_RejectedBalanceForces"=w665:T23)
        n181 = Bundle By Name(cluster=w665, "Timestamp"=w664, "XForces[12]"=w663, "YForces[100]"=w662, "ZForces[156]"=w661, "Fx"=w660, "Fy"=w659, "Fz"=w658, "Mx"=w657, "My"=w656, "Mz"=w655, "ForceMagnitude"=w654) -> (w652:T23)
        n182 = Bundle By Name(cluster=w653, "logevent_RejectedBalanceForces"=w652) -> (w651:T1)
      }
      event User Event {
        n183 = event-data() -> ("Timestamp"=w671:dbl, "SecondaryCylinderForces[112]"=w670:i32[], "PrimaryCylinderForces[156]"=w669:i32[])  [unwired: 1 in, 4 out]
        n184 = Unbundle By Name(w668) -> ("logevent_RejectedCylinderForces"=w672:T24)
        n185 = Bundle By Name(cluster=w672, "Timestamp"=w671, "SecondaryCylinderForces[112]"=w670, "PrimaryCylinderForces[156]"=w669) -> (w667:T24)
        n186 = Bundle By Name(cluster=w668, "logevent_RejectedCylinderForces"=w667) -> (w666:T1)
      }
      event User Event {
        n187 = event-data() -> ("Timestamp"=w686:dbl, "XForces[12]"=w685:sgl[], "YForces[100]"=w684:sgl[], "ZForces[156]"=w683:sgl[], "Fx"=w682:sgl, "Fy"=w681:sgl, "Fz"=w680:sgl, "Mx"=w679:sgl, "My"=w678:sgl, "Mz"=w677:sgl, "ForceMagnitude"=w676:sgl)  [unwired: 1 in, 4 out]
        n188 = Unbundle By Name(w675) -> ("logevent_RejectedElevationForces"=w687:T25)
        n189 = Bundle By Name(cluster=w687, "Timestamp"=w686, "XForces[12]"=w685, "YForces[100]"=w684, "ZForces[156]"=w683, "Fx"=w682, "Fy"=w681, "Fz"=w680, "Mx"=w679, "My"=w678, "Mz"=w677, "ForceMagnitude"=w676) -> (w674:T25)
        n190 = Bundle By Name(cluster=w675, "logevent_RejectedElevationForces"=w674) -> (w673:T1)
      }
      event User Event {
        n191 = event-data() -> ("Timestamp"=w701:dbl, "XForces[12]"=w700:sgl[], "YForces[100]"=w699:sgl[], "ZForces[156]"=w698:sgl[], "Fx"=w697:sgl, "Fy"=w696:sgl, "Fz"=w695:sgl, "Mx"=w694:sgl, "My"=w693:sgl, "Mz"=w692:sgl, "ForceMagnitude"=w691:sgl)  [unwired: 1 in, 4 out]
        n192 = Unbundle By Name(w690) -> ("logevent_RejectedForces"=w702:T26)
        n193 = Bundle By Name(cluster=w702, "Timestamp"=w701, "XForces[12]"=w700, "YForces[100]"=w699, "ZForces[156]"=w698, "Fx"=w697, "Fy"=w696, "Fz"=w695, "Mx"=w694, "My"=w693, "Mz"=w692, "ForceMagnitude"=w691) -> (w689:T26)
        n194 = Bundle By Name(cluster=w690, "logevent_RejectedForces"=w689) -> (w688:T1)
      }
      event User Event {
        n195 = event-data() -> ("Timestamp"=w706:dbl, "XForces[12]"=w707:sgl[], "YForces[100]"=w708:sgl[], "ZForces[156]"=w709:sgl[], "Fx"=w710:sgl, "Fy"=w711:sgl, "Fz"=w712:sgl, "Mx"=w713:sgl, "My"=w714:sgl, "Mz"=w715:sgl, "ForceMagnitude"=w716:sgl)  [unwired: 1 in, 4 out]
        n196 = Unbundle By Name(w705) -> ("logevent_RejectedOffsetForces"=w717:T27)
        n197 = Bundle By Name(cluster=w717, "Timestamp"=w706, "XForces[12]"=w707, "YForces[100]"=w708, "ZForces[156]"=w709, "Fx"=w710, "Fy"=w711, "Fz"=w712, "Mx"=w713, "My"=w714, "Mz"=w715, "ForceMagnitude"=w716) -> (w704:T27)
        n198 = Bundle By Name(cluster=w705, "logevent_RejectedOffsetForces"=w704) -> (w703:T1)
      }
      event User Event {
        n199 = event-data() -> ("Timestamp"=w731:dbl, "XForces[12]"=w730:sgl[], "YForces[100]"=w729:sgl[], "ZForces[156]"=w728:sgl[], "Fx"=w727:sgl, "Fy"=w726:sgl, "Fz"=w725:sgl, "Mx"=w724:sgl, "My"=w723:sgl, "Mz"=w722:sgl, "ForceMagnitude"=w721:sgl)  [unwired: 1 in, 4 out]
        n200 = Unbundle By Name(w720) -> ("logevent_RejectedThermalForces"=w732:T29)
        n201 = Bundle By Name(cluster=w732, "Timestamp"=w731, "XForces[12]"=w730, "YForces[100]"=w729, "ZForces[156]"=w728, "Fx"=w727, "Fy"=w726, "Fz"=w725, "Mx"=w724, "My"=w723, "Mz"=w722, "ForceMagnitude"=w721) -> (w719:T29)
        n202 = Bundle By Name(cluster=w720, "logevent_RejectedThermalForces"=w719) -> (w718:T1)
      }
      event User Event {
        n203 = event-data() -> ("Timestamp"=w746:dbl, "XForces[12]"=w745:sgl[], "YForces[100]"=w744:sgl[], "ZForces[156]"=w743:sgl[], "Fx"=w742:sgl, "Fy"=w741:sgl, "Fz"=w740:sgl, "Mx"=w739:sgl, "My"=w738:sgl, "Mz"=w737:sgl, "ForceMagnitude"=w736:sgl)  [unwired: 1 in, 4 out]
        n204 = Unbundle By Name(w735) -> ("logevent_RejectedVelocityForces"=w747:T30)
        n205 = Bundle By Name(cluster=w747, "Timestamp"=w746, "XForces[12]"=w745, "YForces[100]"=w744, "ZForces[156]"=w743, "Fx"=w742, "Fy"=w741, "Fz"=w740, "Mx"=w739, "My"=w738, "Mz"=w737, "ForceMagnitude"=w736) -> (w734:T30)
        n206 = Bundle By Name(cluster=w735, "logevent_RejectedVelocityForces"=w734) -> (w733:T1)
      }
      event User Event {
        n207 = event-data() -> ("Timestamp"=w784:dbl, "AnyWarning"=w783:bool, "AnySafetyLimitWarning"=w782:bool, "SafetyLimitWarning[156]"=w781:bool[], "XMomentWarning"=w780:bool, "YMomentWarning"=w779:bool, "ZMomentWarning"=w778:bool, "AnyNearNeighborWarning"=w777:bool, "NearNeighborWarning[156]"=w776:bool[], "MagnitudeWarning"=w775:bool, "AnyFarNeighborWarning"=w774:bool, "FarNeighborWarning[156]"=w773:bool[], "AnyElevationForceWarning"=w772:bool, "ElevationForceWarning[156]"=w771:bool[], "AnyAzimuthForceWarning"=w770:bool, "AzimuthForceWarning[156]"=w769:bool[], "AnyThermalForceWarning"=w768:bool, "ThermalForceWarning[156]"=w767:bool[], "AnyBalanceForceWarning"=w766:bool, "BalanceForceWarning[156]"=w765:bool[], "AnyAccelerationForceWarning"=w764:bool, "AccelerationForceWarning[156]"=w763:bool[], "ActiveOpticNetForceWarning"=w762:bool, "AnyActiveOpticForceWarning"=w761:bool, "ActiveOpticForceWarning[156]"=w760:bool[], "AnyStaticForceWarning"=w759:bool, "StaticForceWarning[156]"=w758:bool[], "AberrationNetForceWarning"=w757:bool, "AnyAberrationForceWarning"=w756:bool, "AberrationForceWarning[156]"=w755:bool[], "AnyOffsetForceWarning"=w754:bool, "OffsetForceWarning[156]"=w753:bool[], "AnyVelocityForceWarning"=w752:bool, "VelocityForceWarning[156]"=w751:bool[], "AnyForceWarning"=w750:bool, "ForceWarning[156]"=w749:bool[], "priority"=w748:i32)  [unwired: 1 in, 4 out]
        n208 = Unbundle By Name(w787) -> ("logevent_ForceSetpointWarning"=w788:T31)
        n209 = Bundle By Name(cluster=w788, "Timestamp"=w784, "AnyWarning"=w783, "AnySafetyLimitWarning"=w782, "SafetyLimitWarning[156]"=w781, "XMomentWarning"=w780, "YMomentWarning"=w779, "ZMomentWarning"=w778, "AnyNearNeighborWarning"=w777, "NearNeighborWarning[156]"=w776, "MagnitudeWarning"=w775, "AnyFarNeighborWarning"=w774, "FarNeighborWarning[156]"=w773, "AnyElevationForceWarning"=w772, "ElevationForceWarning[156]"=w771, "AnyAzimuthForceWarning"=w770, "AzimuthForceWarning[156]"=w769, "AnyThermalForceWarning"=w768, "ThermalForceWarning[156]"=w767, "AnyBalanceForceWarning"=w766, "BalanceForceWarning[156]"=w765, "AnyAccelerationForceWarning"=w764, "AccelerationForceWarning[156]"=w763, "ActiveOpticNetForceWarning"=w762, "AnyActiveOpticForceWarning"=w761, "ActiveOpticForceWarning[156]"=w760, "AnyStaticForceWarning"=w759, "StaticForceWarning[156]"=w758, "AberrationNetForceWarning"=w757, "AnyAberrationForceWarning"=w756, "AberrationForceWarning[156]"=w755, "AnyOffsetForceWarning"=w754, "OffsetForceWarning[156]"=w753, "AnyVelocityForceWarning"=w752, "VelocityForceWarning[156]"=w751, "AnyForceWarning"=w750, "ForceWarning[156]"=w749, "priority"=w748) -> (w786:T31)
        n210 = Bundle By Name(cluster=w787, "logevent_ForceSetpointWarning"=w786) -> (w785:T1)
      }
    }
    "stop" <- w272
    n211 = local write "FA Data And Events"(w273) -> ()
  }
  n212 = control-ref of="This VI"() -> (w60:refnum<vi>)
  n213 = call "Close References.vi"("error in (no error)"=w14, "VI Refnum"=w60, "Variant"=w13) -> ("error out"=w12:errorcluster)  [unwired: 8 in]
  n214 = Not A Number/Path/Refnum?(number/path/refnum=w58) -> (NaN/Path/Refnum?=w59:bool)
  n215 = case shown="True" w59 {
    tunnel: w58 -> [_ w792]
    tunnel: w12 -> [w789 w791]
    tunnel: [w789 w790] -> w57
    frame False {
    }
    frame True {
      n216 = Unregister For Events(event registration refnum=w792, error in=w791) -> (error out=w790:errorcluster)
    }
  }
  n217 = call <vilib>:"Simple Error Handler.vi"("error in (no error)"=w57) -> ()  [unwired: 4 in, 5 out]
